vi "总磷总氮通讯.vi"() -> ()   [LabVIEW 2016, in "斯坦道总磷总氮.lvlib"]
uses:
  <vilib>/Plasmionique/MB Master/MB_Master_Serial/MB_Master_Serial.lvclass
  C:/Program Files (x86)/National Instruments/LabVIEW 2016/vi.lib/Plasmionique/MB Master/MB_Master/MB_Master.lvclass
  <vilib>/Plasmionique/MB Master/MB_Master_TCP/MB_Master_TCP.lvclass
  <vilib>/Utility/config.llb/Write Key (Boolean).vi
  <vilib>/Utility/config.llb/Write Key (String).vi
  <vilib>/Plasmionique/MB Master/MB_Master/MB_Master.lvclass
  <vilib>/Utility/config.llb/NI_LVConfig.lvlib
  <vilib>/Plasmionique/MB Master/MB Master.lvlib
  <vilib>/ptbypt/NI_PtbyPt.lvlib
panel:
  out "启用":bool=TRUE
  out "氨氮状态告警区":u16[](array[numeric])
  out "氨氮测量数据区":u16[](array[numeric])
  out "COD测量数据区":u16[](array[numeric])
  out "COD状态告警区":u16[](array[numeric])
  out "总氮测量数据区":u16[](array[numeric])
  out "总氮状态告警区":u16[](array[numeric])
  out "总磷状态告警区":u16[](array[numeric])
  out "总磷测量数据区":u16[](array[numeric])
  out "状态告警区":T1 {"告警代码" items=["无告警", "缺试剂告警", "缺水样告警", "缺蒸馏水告警", "缺标液告警", "仪表漏液告警", "标定异常告警", "超量程告警", "加热异常", "低试剂预警", "超上限告警", "超下限告警", "仪表内部其他异常", "滴定异常告警", "电极异常告警", "量程切换告警", "参数设置告警", "PH电极电位异常", "电导率电极异常", "浊度光度异常", "溶解氧电极异常", "溶解氧光强异常", "温度异常告警", "PH异常告警", "溶解氧异常告警", "电导率异常告警", "浊度异常告警", "叶绿素异常告警", "藻密度异常告警", "蓝绿藻异常告警", "ORP异常告警", "氨氮异常告警", "清洁刷异常告警", "SD卡异常告警", "蓝牙异常告警", "Wifi异常告警", "流程异常告警"]; "故障代码" items=["无故障", "电机故障", "温度故障", "通讯故障", "滴定故障"]}
  out "测量数据区":T2 {"单位" items=["ug/L", "mg/L", "ppm", "mg/m3", "cm", "ppb", "ug/m3", "%", "nmol/mol", "umol/mol", "MPN/L", "MPN/100ml", "ng/m3", "NTU", "无量纲", "ms/cm", "us/cm", "℃", "mV", "万个/L"]}
  out "status":bool
  out "关键参数区":T3
  in  "读关键参数区":bool
  in  "读状态告警区":bool
  in  "读测量数据区":bool
  in  "站号":u16(ring) items=["总磷"=1, "氨氮"=3]
  in  "停止":bool
  in  "启动":bool
  in  "控制命令":u16(ring) items=["启动测量"=1, "标样核查"=2, "零点核查"=3, "跨度核查"=4, "空白测试"=5, "平行样测试"=6, "加标回收"=7, "空白校准"=8, "标样校准"=9, "初始化（清洗）"=10, "停止测试"=11, "仪器重启"=12, "校时"=13, "模式设置"=14, "测量间隔设置"=15]
  in  "控制命令参数":u16[](array[numeric]) format="%04xH"
  in  "VISA Resource":refnum<visa-resource-name>
  in  "启用模块":bool
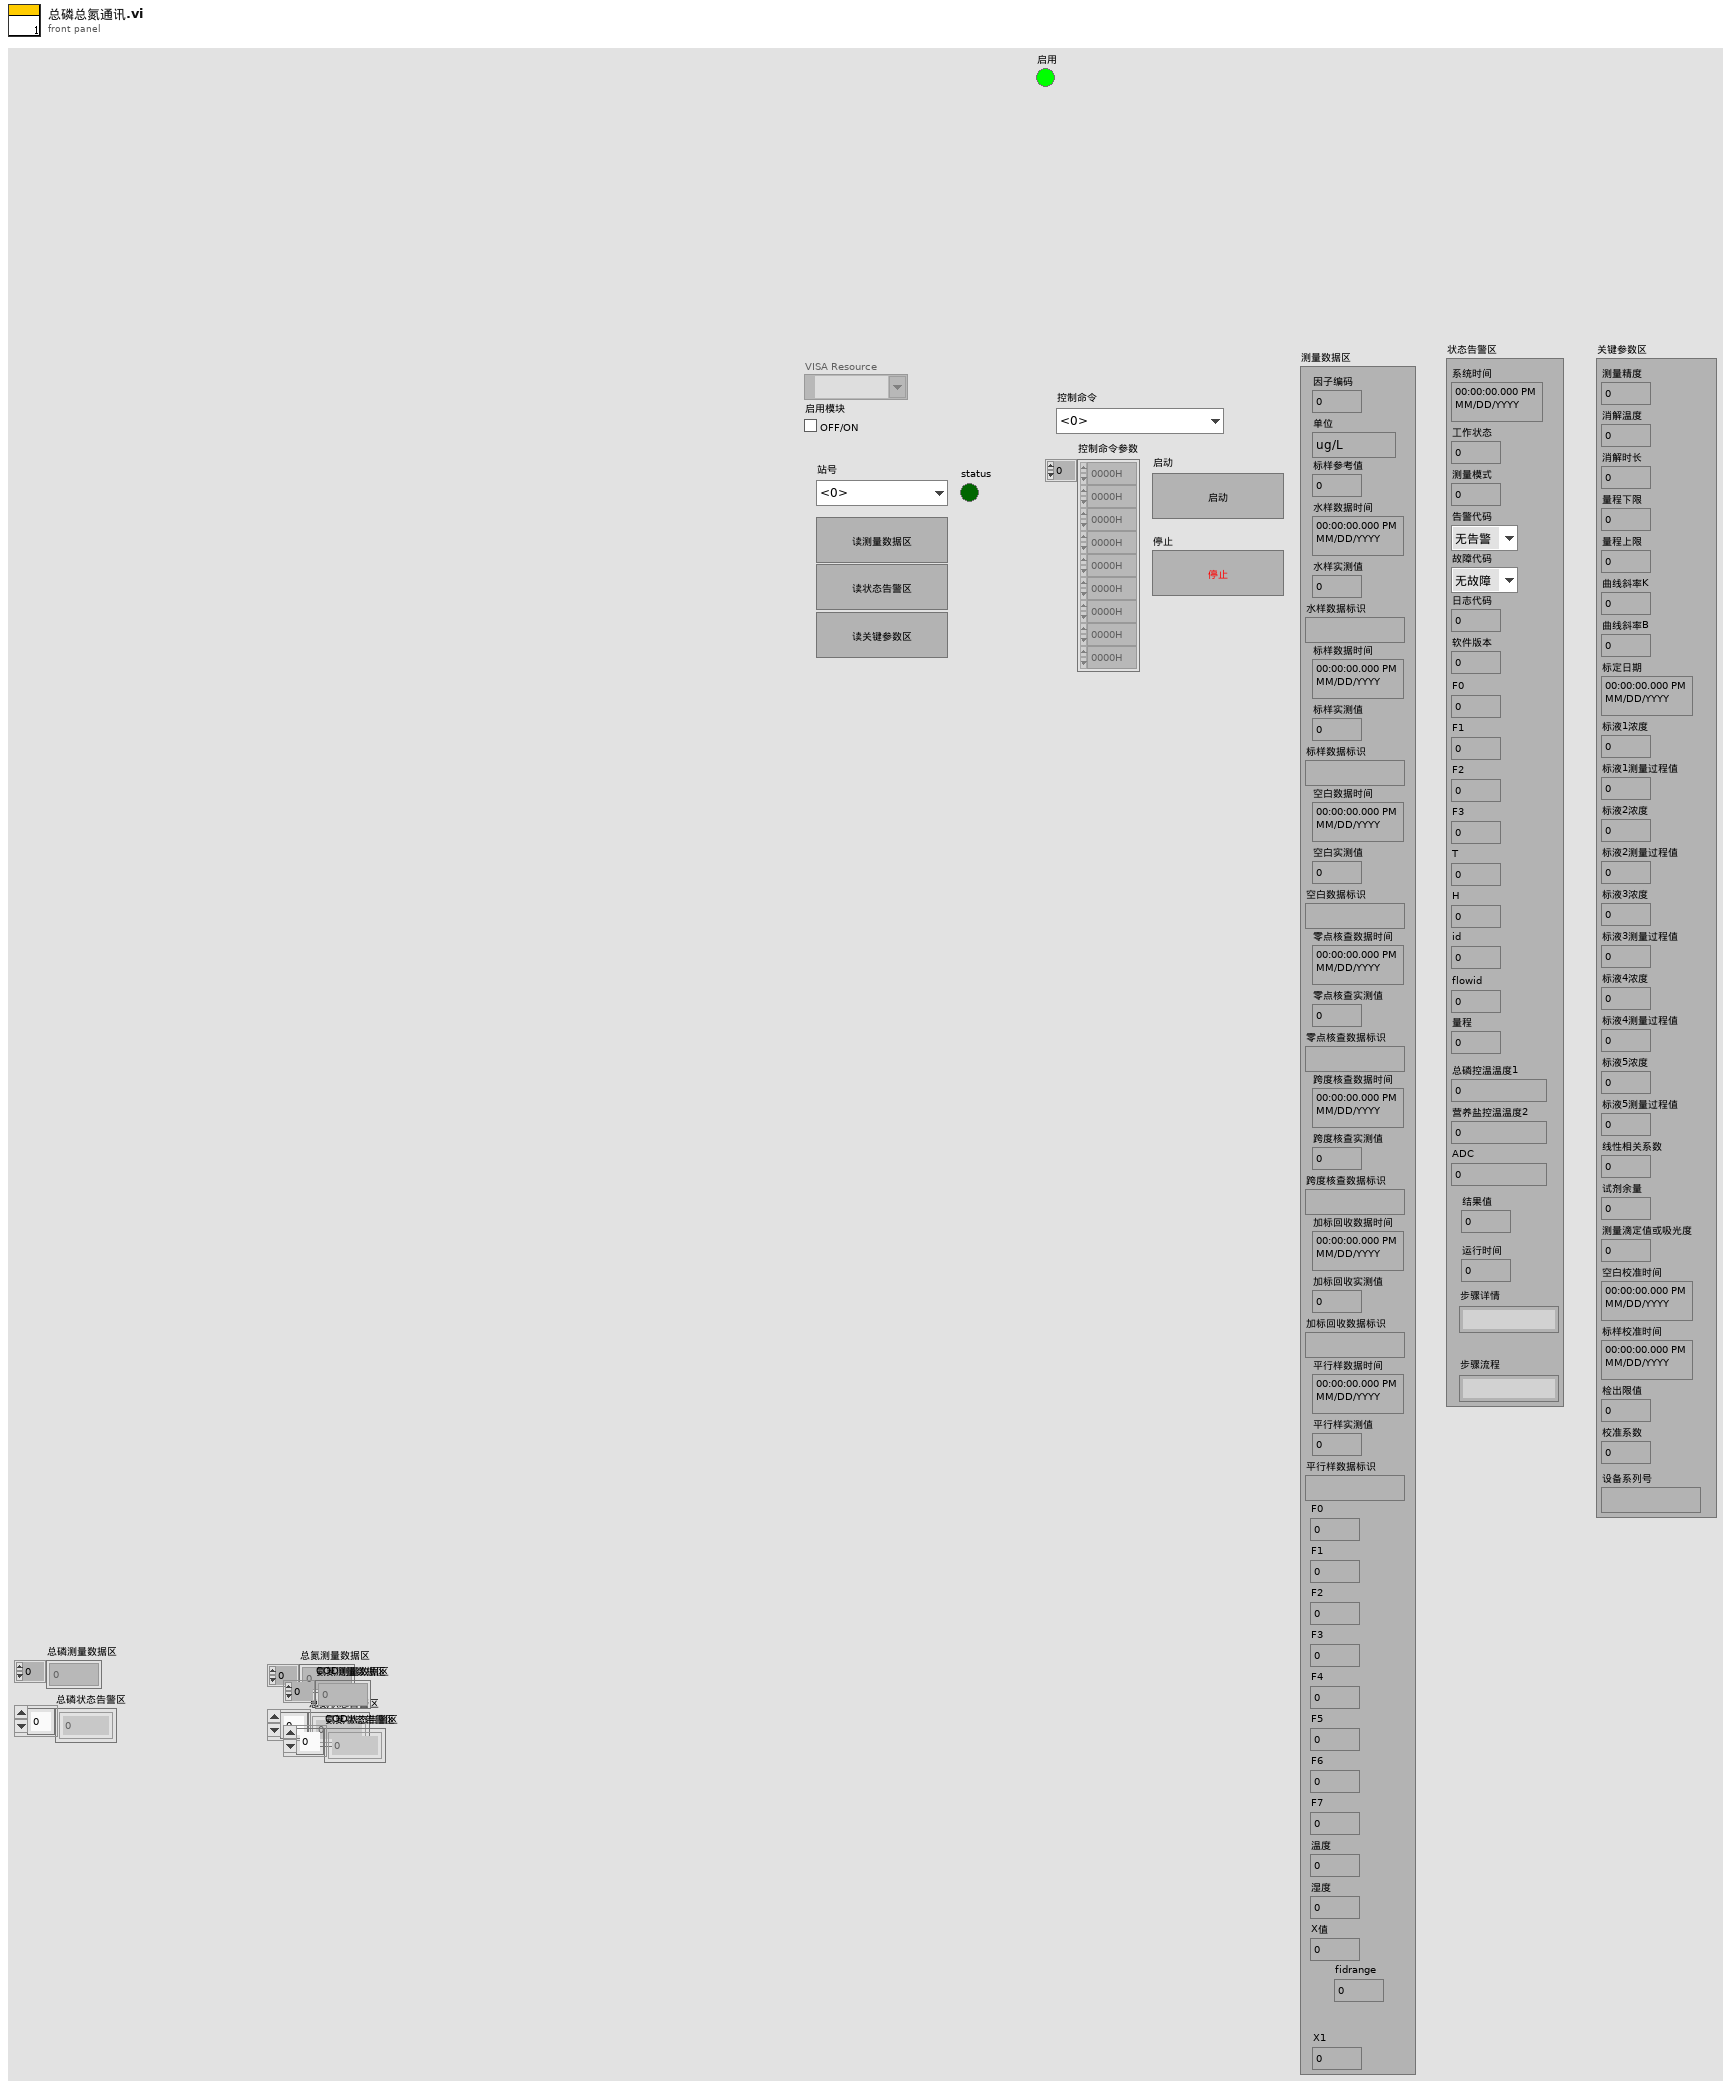
[diagram p1: front panel]
types:
  T1 = cluster{"系统时间":timestamp, "工作状态":u16, "测量模式":u16, "告警代码":u16, "故障代码":u16, "日志代码":u16, "软件版本":u16, "F0":sgl, "F1":sgl, "F2":sgl, "F3":sgl, "T":sgl, "H":sgl, "id":u16, "flowid":u16, "量程":u16, "总磷控温温度1":sgl, "营养盐控温温度2":sgl, "ADC":sgl, "结果值":sgl, "运行时间":u16, "步骤详情":string, "步骤流程":string}
  T2 = cluster{"因子编码":u32, "单位":u16, "标样参考值":sgl, "水样数据时间":timestamp, "水样实测值":sgl, "水样数据标识":string, "标样数据时间":timestamp, "标样实测值":sgl, "标样数据标识":string, "空白数据时间":timestamp, "空白实测值":sgl, "空白数据标识":string, "零点核查数据时间":timestamp, "零点核查实测值":sgl, "零点核查数据标识":string, "跨度核查数据时间":timestamp, "跨度核查实测值":sgl, "跨度核查数据标识":string, "加标回收数据时间":timestamp, "加标回收实测值":sgl, "加标回收数据标识":string, "平行样数据时间":timestamp, "平行样实测值":sgl, "平行样数据标识":string, "F0":sgl, "F1":sgl, "F2":sgl, "F3":sgl, "F4":sgl, "F5":sgl, "F6":sgl, "F7":sgl, "温度":sgl, "湿度":sgl, "X值":sgl, "fidrange":u16, "X1":sgl}
  T3 = cluster{"测量精度":u16, "消解温度":u16, "消解时长":u16, "量程下限":sgl, "量程上限":sgl, "曲线斜率K":sgl, "曲线斜率B":sgl, "标定日期":timestamp, "标液1浓度":sgl, "标液1测量过程值":sgl, "标液2浓度":sgl, "标液2测量过程值":sgl, "标液3浓度":sgl, "标液3测量过程值":sgl, "标液4浓度":sgl, "标液4测量过程值":sgl, "标液5浓度":sgl, "标液5测量过程值":sgl, "线性相关系数":sgl, "试剂余量":u32, "测量滴定值或吸光度":sgl, "空白校准时间":timestamp, "标样校准时间":timestamp, "检出限值":sgl, "校准系数":sgl, "设备系列号":string}
  T4 = cluster{"系统时间":timestamp, "工作状态":u16, "测量模式":enum16{"待机", "连续模式", "周期模式", "定点模式", "受控模式", "手动模式"}, "告警代码":u16, "故障代码":u16, "日志代码":u16, "软件版本":u16, "F0":sgl, "F1":sgl, "F2":sgl, "F3":sgl, "T":sgl, "H":sgl, "id":u16, "flowid":u16, "量程":u16, "总磷控温温度1":sgl, "营养盐控温温度2":sgl, "ADC":sgl}
  T5 = cluster{"因子编码":u32, "单位":u16, "标样参考值":sgl, "水样数据时间":timestamp, "水样实测值":sgl, "水样数据标识":string, "标样数据时间":timestamp, "标样实测值":sgl, "标样数据标识":string, "空白数据时间":timestamp, "空白实测值":sgl, "空白数据标识":string, "零点核查数据时间":timestamp, "零点核查实测值":sgl, "零点核查数据标识":string, "跨度核查数据时间":timestamp, "跨度核查实测值":sgl, "跨度核查数据标识":string, "加标回收数据时间":timestamp, "加标回收实测值":sgl, "加标回收数据标识":string, "平行样数据时间":timestamp, "平行样实测值":sgl, "平行样数据标识":string, "F0":sgl, "F1":sgl, "F2":sgl, "F3":sgl, "F4":sgl, "F5":sgl, "F6":sgl, "F7":sgl, "温度":sgl, "湿度":sgl, "X值":sgl, "fidrange":u16, "X1值":sgl}
  T6 = cluster{"测量精度":u16, "消解温度":u16, "消解时长":u16, "量程下限":sgl, "量程上限":sgl, "曲线斜率K":sgl, "曲线斜率B":sgl, "标定日期":timestamp, "标液1浓度":sgl, "标液1测量过程值":sgl, "标液2浓度":sgl, "标液2测量过程值":sgl, "标液3浓度":sgl, "标液3测量过程值":sgl, "标液4浓度":sgl, "标液4测量过程值":sgl, "标液5浓度":sgl, "标液5测量过程值":sgl, "线性相关系数":sgl, "试剂余量":u32, "测量滴定值或吸光度":sgl, "空白校准时间":timestamp, "标样校准时间":timestamp, "检出限值":sgl, "校准系数":sgl, "设备系列号":string}[]
  T7 = cluster{"系统时间":timestamp, "工作状态":u16, "测量模式":enum16{"待机", "连续模式", "周期模式", "定点模式", "受控模式", "手动模式"}, "告警代码":u16, "故障代码":u16, "日志代码":u16, "软件版本":u16, "F0":sgl, "F1":sgl, "F2":sgl, "F3":sgl, "T":sgl, "H":sgl, "id":u16, "flowid":u16, "量程":u16, "总磷控温温度1":sgl, "营养盐控温温度2":sgl, "ADC":sgl}[]
  T8 = cluster{"因子编码":u32, "单位":u16, "标样参考值":sgl, "水样数据时间":timestamp, "水样实测值":sgl, "水样数据标识":string, "标样数据时间":timestamp, "标样实测值":sgl, "标样数据标识":string, "空白数据时间":timestamp, "空白实测值":sgl, "空白数据标识":string, "零点核查数据时间":timestamp, "零点核查实测值":sgl, "零点核查数据标识":string, "跨度核查数据时间":timestamp, "跨度核查实测值":sgl, "跨度核查数据标识":string, "加标回收数据时间":timestamp, "加标回收实测值":sgl, "加标回收数据标识":string, "平行样数据时间":timestamp, "平行样实测值":sgl, "平行样数据标识":string, "F0":sgl, "F1":sgl, "F2":sgl, "F3":sgl, "F4":sgl, "F5":sgl, "F6":sgl, "F7":sgl, "温度":sgl, "湿度":sgl, "X值":sgl, "fidrange":u16, "X1值":sgl}[]
  T9 = enum16{"", "CODMn", "PH", "氨氮", "总氮", "总磷", "CODCr", "电导率", "水温", "溶解氧", "浊度", "叶绿素", "藻密度", "ORP"}
  T10 = typedef "CODCr交互.ctl" = cluster{"状态告警区":cluster{"系统时间":timestamp, "工作状态":u16, "测量模式":enum16{"待机", "连续模式", "周期模式", "定点模式", "受控模式", "手动模式"}, "告警代码":u16, "故障代码":u16, "日志代码":u16, "软件版本":u16, "F0":sgl, "F1":sgl, "F2":sgl, "F3":sgl, "T":sgl, "H":sgl, "id":u16, "flowid":u16, "量程":u16, "总磷控温温度1":sgl, "营养盐控温温度2":sgl, "ADC":sgl}, "平台试剂余量百分比":sgl, "关键参数":cluster{"测量量程":dbl, "测量精度":dbl, "测量间隔":dbl, "消解温度":dbl, "消解时长":dbl, "空白校准时间":timestamp, "曲线截距":dbl, "曲线斜率":dbl, "测量检出限":dbl, "测量信号值":dbl, "线性相关系数":dbl, "二次多项式系数":dbl, "标样校准时间":timestamp, "稀释倍数":dbl, "三项式系数":dbl, "空白标定系数":dbl, "量程系数":dbl, "F0/ORPA":dbl, "F1/ORPB":dbl, "F2/ORPK":dbl, "F3":dbl, "F4":dbl, "F5":dbl, "F6":dbl, "F7":dbl, "X0/滴定数":dbl, "量程":dbl}, "关键参数改变":bool, "校准信息":cluster{"低标液1浓度":dbl, "低标液1信号值":dbl, "低标液1启用":u16, "低标液2浓度":dbl, "低标液2信号值":dbl, "低标液2启用":u16, "低标液3浓度":dbl, "低标液3信号值":dbl, "低标液3启用":u16, "低标液4浓度":dbl, "低标液4信号值":dbl, "低标液4启用":u16, "低标液5浓度":dbl, "低标液5信号值":dbl, "低标液5启用":u16, "高标液1浓度":dbl, "高标液1信号值":dbl, "高标液1启用":u16, "高标液2浓度":dbl, "高标液2信号值":dbl, "高标液2启用":u16, "高标液3浓度":dbl, "高标液3信号值":dbl, "高标液3启用":u16, "高标液4浓度":dbl, "高标液4信号值":dbl, "高标液4启用":u16, "高标液5浓度":dbl, "高标液5信号值":dbl, "高标液5启用":u16, "低斜率":dbl, "低截距":dbl, "低二次多项式系数":dbl, "低线性相关系数":dbl, "高斜率":dbl, "高截距":dbl, "高二次多项式系数":dbl, "高线性相关系数":dbl}, "校准信息改变":bool, "固件版本号":string}
  T11 = typedef "氨氮交互.ctl" = cluster{"状态告警区":cluster{"系统时间":timestamp, "工作状态":u16, "测量模式":enum16{"待机", "连续模式", "周期模式", "定点模式", "受控模式", "手动模式"}, "告警代码":u16, "故障代码":u16, "日志代码":u16, "软件版本":u16, "F0":sgl, "F1":sgl, "F2":sgl, "F3":sgl, "T":sgl, "H":sgl, "id":u16, "flowid":u16, "量程":u16, "总磷控温温度1":sgl, "营养盐控温温度2":sgl, "ADC":sgl}, "平台试剂余量百分比":sgl, "关键参数":cluster{"测量量程":dbl, "测量精度":dbl, "测量间隔":dbl, "消解温度":dbl, "消解时长":dbl, "空白校准时间":timestamp, "曲线截距":dbl, "曲线斜率":dbl, "测量检出限":dbl, "测量信号值":dbl, "线性相关系数":dbl, "二次多项式系数":dbl, "标样校准时间":timestamp, "稀释倍数":dbl, "三项式系数":dbl, "空白标定系数":dbl, "量程系数":dbl, "F0/ORPA":dbl, "F1/ORPB":dbl, "F2/ORPK":dbl, "F3":dbl, "F4":dbl, "F5":dbl, "F6":dbl, "F7":dbl, "X0/滴定数":dbl, "量程":dbl}, "关键参数改变":bool, "校准信息":cluster{"低标液1浓度":dbl, "低标液1信号值":dbl, "低标液1启用":u16, "低标液2浓度":dbl, "低标液2信号值":dbl, "低标液2启用":u16, "低标液3浓度":dbl, "低标液3信号值":dbl, "低标液3启用":u16, "低标液4浓度":dbl, "低标液4信号值":dbl, "低标液4启用":u16, "低标液5浓度":dbl, "低标液5信号值":dbl, "低标液5启用":u16, "高标液1浓度":dbl, "高标液1信号值":dbl, "高标液1启用":u16, "高标液2浓度":dbl, "高标液2信号值":dbl, "高标液2启用":u16, "高标液3浓度":dbl, "高标液3信号值":dbl, "高标液3启用":u16, "高标液4浓度":dbl, "高标液4信号值":dbl, "高标液4启用":u16, "高标液5浓度":dbl, "高标液5信号值":dbl, "高标液5启用":u16, "低斜率":dbl, "低截距":dbl, "低二次多项式系数":dbl, "低线性相关系数":dbl, "高斜率":dbl, "高截距":dbl, "高二次多项式系数":dbl, "高线性相关系数":dbl}, "校准信息改变":bool, "固件版本号":string}
  T12 = typedef "总氮交互.ctl" = cluster{"状态告警区":cluster{"系统时间":timestamp, "工作状态":u16, "测量模式":enum16{"待机", "连续模式", "周期模式", "定点模式", "受控模式", "手动模式"}, "告警代码":u16, "故障代码":u16, "日志代码":u16, "软件版本":u16, "F0":sgl, "F1":sgl, "F2":sgl, "F3":sgl, "T":sgl, "H":sgl, "id":u16, "flowid":u16, "量程":u16, "总磷控温温度1":sgl, "营养盐控温温度2":sgl, "ADC":sgl}, "平台试剂余量百分比":sgl, "关键参数":cluster{"测量量程":dbl, "测量精度":dbl, "测量间隔":dbl, "消解温度":dbl, "消解时长":dbl, "空白校准时间":timestamp, "曲线截距":dbl, "曲线斜率":dbl, "测量检出限":dbl, "测量信号值":dbl, "线性相关系数":dbl, "二次多项式系数":dbl, "标样校准时间":timestamp, "稀释倍数":dbl, "三项式系数":dbl, "空白标定系数":dbl, "量程系数":dbl, "F0/ORPA":dbl, "F1/ORPB":dbl, "F2/ORPK":dbl, "F3":dbl, "F4":dbl, "F5":dbl, "F6":dbl, "F7":dbl, "X0/滴定数":dbl, "量程":dbl}, "关键参数改变":bool, "校准信息":cluster{"低标液1浓度":dbl, "低标液1信号值":dbl, "低标液1启用":u16, "低标液2浓度":dbl, "低标液2信号值":dbl, "低标液2启用":u16, "低标液3浓度":dbl, "低标液3信号值":dbl, "低标液3启用":u16, "低标液4浓度":dbl, "低标液4信号值":dbl, "低标液4启用":u16, "低标液5浓度":dbl, "低标液5信号值":dbl, "低标液5启用":u16, "高标液1浓度":dbl, "高标液1信号值":dbl, "高标液1启用":u16, "高标液2浓度":dbl, "高标液2信号值":dbl, "高标液2启用":u16, "高标液3浓度":dbl, "高标液3信号值":dbl, "高标液3启用":u16, "高标液4浓度":dbl, "高标液4信号值":dbl, "高标液4启用":u16, "高标液5浓度":dbl, "高标液5信号值":dbl, "高标液5启用":u16, "低斜率":dbl, "低截距":dbl, "低二次多项式系数":dbl, "低线性相关系数":dbl, "高斜率":dbl, "高截距":dbl, "高二次多项式系数":dbl, "高线性相关系数":dbl}, "校准信息改变":bool, "固件版本号":string}
  T13 = typedef "总磷交互.ctl" = cluster{"状态告警区":cluster{"系统时间":timestamp, "工作状态":u16, "测量模式":enum16{"待机", "连续模式", "周期模式", "定点模式", "受控模式", "手动模式"}, "告警代码":u16, "故障代码":u16, "日志代码":u16, "软件版本":u16, "F0":sgl, "F1":sgl, "F2":sgl, "F3":sgl, "T":sgl, "H":sgl, "id":u16, "flowid":u16, "量程":u16, "总磷控温温度1":sgl, "营养盐控温温度2":sgl, "ADC":sgl}, "平台试剂余量百分比":sgl, "关键参数":cluster{"测量量程":dbl, "测量精度":dbl, "测量间隔":dbl, "消解温度":dbl, "消解时长":dbl, "空白校准时间":timestamp, "曲线截距":dbl, "曲线斜率":dbl, "测量检出限":dbl, "测量信号值":dbl, "线性相关系数":dbl, "二次多项式系数":dbl, "标样校准时间":timestamp, "稀释倍数":dbl, "三项式系数":dbl, "空白标定系数":dbl, "量程系数":dbl, "F0/ORPA":dbl, "F1/ORPB":dbl, "F2/ORPK":dbl, "F3":dbl, "F4":dbl, "F5":dbl, "F6":dbl, "F7":dbl, "X0/滴定数":dbl, "量程":dbl}, "关键参数改变":bool, "校准信息":cluster{"低标液1浓度":dbl, "低标液1信号值":dbl, "低标液1启用":u16, "低标液2浓度":dbl, "低标液2信号值":dbl, "低标液2启用":u16, "低标液3浓度":dbl, "低标液3信号值":dbl, "低标液3启用":u16, "低标液4浓度":dbl, "低标液4信号值":dbl, "低标液4启用":u16, "低标液5浓度":dbl, "低标液5信号值":dbl, "低标液5启用":u16, "高标液1浓度":dbl, "高标液1信号值":dbl, "高标液1启用":u16, "高标液2浓度":dbl, "高标液2信号值":dbl, "高标液2启用":u16, "高标液3浓度":dbl, "高标液3信号值":dbl, "高标液3启用":u16, "高标液4浓度":dbl, "高标液4信号值":dbl, "高标液4启用":u16, "高标液5浓度":dbl, "高标液5信号值":dbl, "高标液5启用":u16, "低斜率":dbl, "低截距":dbl, "低二次多项式系数":dbl, "低线性相关系数":dbl, "高斜率":dbl, "高截距":dbl, "高二次多项式系数":dbl, "高线性相关系数":dbl}, "校准信息改变":bool, "固件版本号":string}
  T14 = typedef "操作日志字段定义.ctl" = cluster{"时间":timestamp, "参数":string, "日志信息":string, "流程参数":string}
  T15 = typedef "NI_LVConfig.lvlib/Config Data RefNum.ctl" = refnum<k1>
  T16 = enum8{"Enabled", "Disabled", "Disabled and Grayed Out"}
  T17 = cluster{"baud rate (bps)":u32, "stop bits":u16, "parity":u16, "flow control":u16, "timeout":u32, "retries":i32}
  T18 = typedef "工况数据.ctl" = cluster{"time":string, "data":cluster{"ups":cluster{"ups":cluster{"input_voltage":ext, "input_frequency":ext, "output_voltage":ext, "output_current":ext, "output_frequency":ext, "output_active_power":ext, "output_apparent_power":ext, "load_rate":ext, "cabinet_temperature":ext, "battery_voltage":ext, "remaining_battery_capacity":ext, "power_on_status":string, "power_supply_mode":string, "fault":bool, "battery_low_voltage":bool, "mains_supply_abnormality":bool}, "启用":bool}, "air_conditioner":cluster{"air_conditioner":cluster{"cabinet_temperature":ext, "air_supply_temperature":ext, "voltage":ext, "current":ext, "compressor_status":string, "Internal_fan_status":string, "external_fan_status":string, "heating_state":string, "refrigeration_state":bool, "high_temperature_alarm":bool, "low_temperature_alarm":bool, "heater_fault":bool, "temperature_sensor_fault":bool, "high_voltage_alarm":bool, "low_voltage_alarm":bool, "refrigeration_start_point":ext, "refrigeration_sensitive_point":ext, "heating_start_point":ext, "heating_sensitive_point":ext, "high_temperature_alarm_point":ext, "low_temperature_alarm_point":ext}, "启用":bool}, "smoke_sensor":cluster{"smoke_sensor":cluster{"trigger_alarm":bool}, "启用":bool}, "water_immersion_sensor":cluster{"water_immersion_sensor":cluster{"trigger_alarm":bool}, "启用":bool}, "temperature_and_humidity_sensor":cluster{"temperature_and_humidity_sensor":cluster{"current_temperature":ext, "current_humidity":ext, "room_temperature_alarm":bool, "humidity_alarm":bool}, "启用":bool}, "gps":cluster{"gps":cluster{"current_longitude":ext, "current_latitude":ext, "launch_longitude":ext, "launch_latitude":ext, "shift_alarm":bool}, "启用":bool}, "solar_controller":cluster{"solar_controller":cluster{"array_voltage":ext, "array_current":ext, "generating_power":ext, "battery_voltage":dbl, "battery_current":ext, "ceiling_voltage":ext, "minimum_voltage":ext, "battery_temperature":ext, "remaining_battery_capacity":ext, "load_voltage":ext, "load_current":ext, "load_power":ext, "equipment_temperature":ext, "accumulated_electricity_consumption_of_the_day":ext, "accumulated_electricity_consumption_of_the_current_month":ext, "accumulated_electricity_consumption_in_the_current_year":ext, "total_accumulated_power_consumption":ext, "accumulated_charging_capacity_of_the_day":ext, "accumulated_charging_amount_of_the_current_month":ext, "accumulated_charging_capacity_of_the_current_year":ext, "total_cumulative_charge":ext}, "启用":bool}, "solar_controller_2":cluster{"solar_controller_2":cluster{"array_voltage":ext, "array_current":ext, "generating_power":ext, "battery_voltage":dbl, "battery_current":ext, "ceiling_voltage":ext, "minimum_voltage":ext, "battery_temperature":ext, "remaining_battery_capacity":ext, "load_voltage":ext, "load_current":ext, "load_power":ext, "equipment_temperature":ext, "accumulated_electricity_consumption_of_the_day":ext, "accumulated_electricity_consumption_of_the_current_month":ext, "accumulated_electricity_consumption_in_the_current_year":ext, "total_accumulated_power_consumption":ext, "accumulated_charging_capacity_of_the_day":ext, "accumulated_charging_amount_of_the_current_month":ext, "accumulated_charging_capacity_of_the_current_year":ext, "total_cumulative_charge":ext}, "启用":bool}, "NH3":cluster{"NH3":cluster{"F0":ext, "F1":ext, "syringe_temperature":ext, "alarm_step":dbl, "X0":ext}, "启用":bool}, "TP":cluster{"TP":cluster{"F0":ext, "F1":ext, "F2":ext, "F3":ext, "digestion_temperature":ext, "constant_temperature":ext, "syringe_temperature":ext, "alarm_step":dbl, "X0":ext}, "启用":bool}, "TN":cluster{"TN":cluster{"F0":ext, "F1":ext, "F2":ext, "F3":ext, "F4":ext, "F5":ext, "F6":ext, "F7":ext, "digestion_temperature":ext, "constant_temperature":ext, "syringe_temperature":ext, "alarm_step":dbl, "X0":ext}, "启用":bool}, "CODMn":cluster{"CODMn":cluster{"temperature_curve":ext[], "titration_curve":ext[], "F0":ext, "F1":ext, "F2":ext, "F3":ext, "F4":ext, "F5":ext, "A":ext, "B":ext, "K":ext}, "启用":bool}, "CODCr":cluster{"CODCr":cluster{"temperature_curve":ext[], "F0":ext, "F1":ext, "reagent_sensor":ext}, "启用":bool}}}
  T19 = cluster{"系统时间":timestamp, "工作状态":u16, "测量模式":enum16{"待机", "连续模式", "周期模式", "定点模式", "受控模式", "手动模式"}, "告警代码":u16, "故障代码":u16, "日志代码":u16, "软件版本":u16, "F0":sgl, "F1":sgl, "F2":sgl, "F3":sgl, "T":sgl, "H":sgl, "id":u16, "flowid":u16, "量程":u16, "总磷控温温度1":sgl, "营养盐控温温度2":sgl, "ADC":sgl, "结果值":sgl, "运行时间":u16, "步骤详情":string, "步骤流程":string}
  T20 = typedef "斯坦道总磷总氮.lvlib/关键参数.ctl" = cluster{"测量量程":sgl, "测量检出限":sgl, "测量精度":sgl, "测量间隔":sgl, "消解温度":sgl, "消解时长":sgl, "三项式系数":sgl, "二次多项式系数":sgl, "曲线斜率":sgl, "曲线截距":sgl, "线性相关系数":sgl, "空白校准时间":timestamp, "标样校准时间":timestamp, "测量信号值":sgl, "稀释倍数":sgl, "空白标定系数":sgl, "量程系数":sgl}
  T21 = cluster{"测量量程":dbl, "测量精度":dbl, "测量间隔":dbl, "消解温度":dbl, "消解时长":dbl, "空白校准时间":timestamp, "曲线截距":dbl, "曲线斜率":dbl, "测量检出限":dbl, "测量信号值":dbl, "线性相关系数":dbl, "二次多项式系数":dbl, "标样校准时间":timestamp, "稀释倍数":dbl, "三项式系数":dbl, "空白标定系数":dbl, "量程系数":dbl, "F0/ORPA":dbl, "F1/ORPB":dbl, "F2/ORPK":dbl, "F3":dbl, "F4":dbl, "F5":dbl, "F6":dbl, "F7":dbl, "X0/滴定数":dbl, "量程":dbl}
  T22 = cluster{"低标液1浓度":dbl, "低标液1信号值":dbl, "低标液1启用":u16, "低标液2浓度":dbl, "低标液2信号值":dbl, "低标液2启用":u16, "低标液3浓度":dbl, "低标液3信号值":dbl, "低标液3启用":u16, "低标液4浓度":dbl, "低标液4信号值":dbl, "低标液4启用":u16, "低标液5浓度":dbl, "低标液5信号值":dbl, "低标液5启用":u16, "高标液1浓度":dbl, "高标液1信号值":dbl, "高标液1启用":u16, "高标液2浓度":dbl, "高标液2信号值":dbl, "高标液2启用":u16, "高标液3浓度":dbl, "高标液3信号值":dbl, "高标液3启用":u16, "高标液4浓度":dbl, "高标液4信号值":dbl, "高标液4启用":u16, "高标液5浓度":dbl, "高标液5信号值":dbl, "高标液5启用":u16, "低斜率":dbl, "低截距":dbl, "低二次多项式系数":dbl, "低线性相关系数":dbl, "高斜率":dbl, "高截距":dbl, "高二次多项式系数":dbl, "高线性相关系数":dbl}
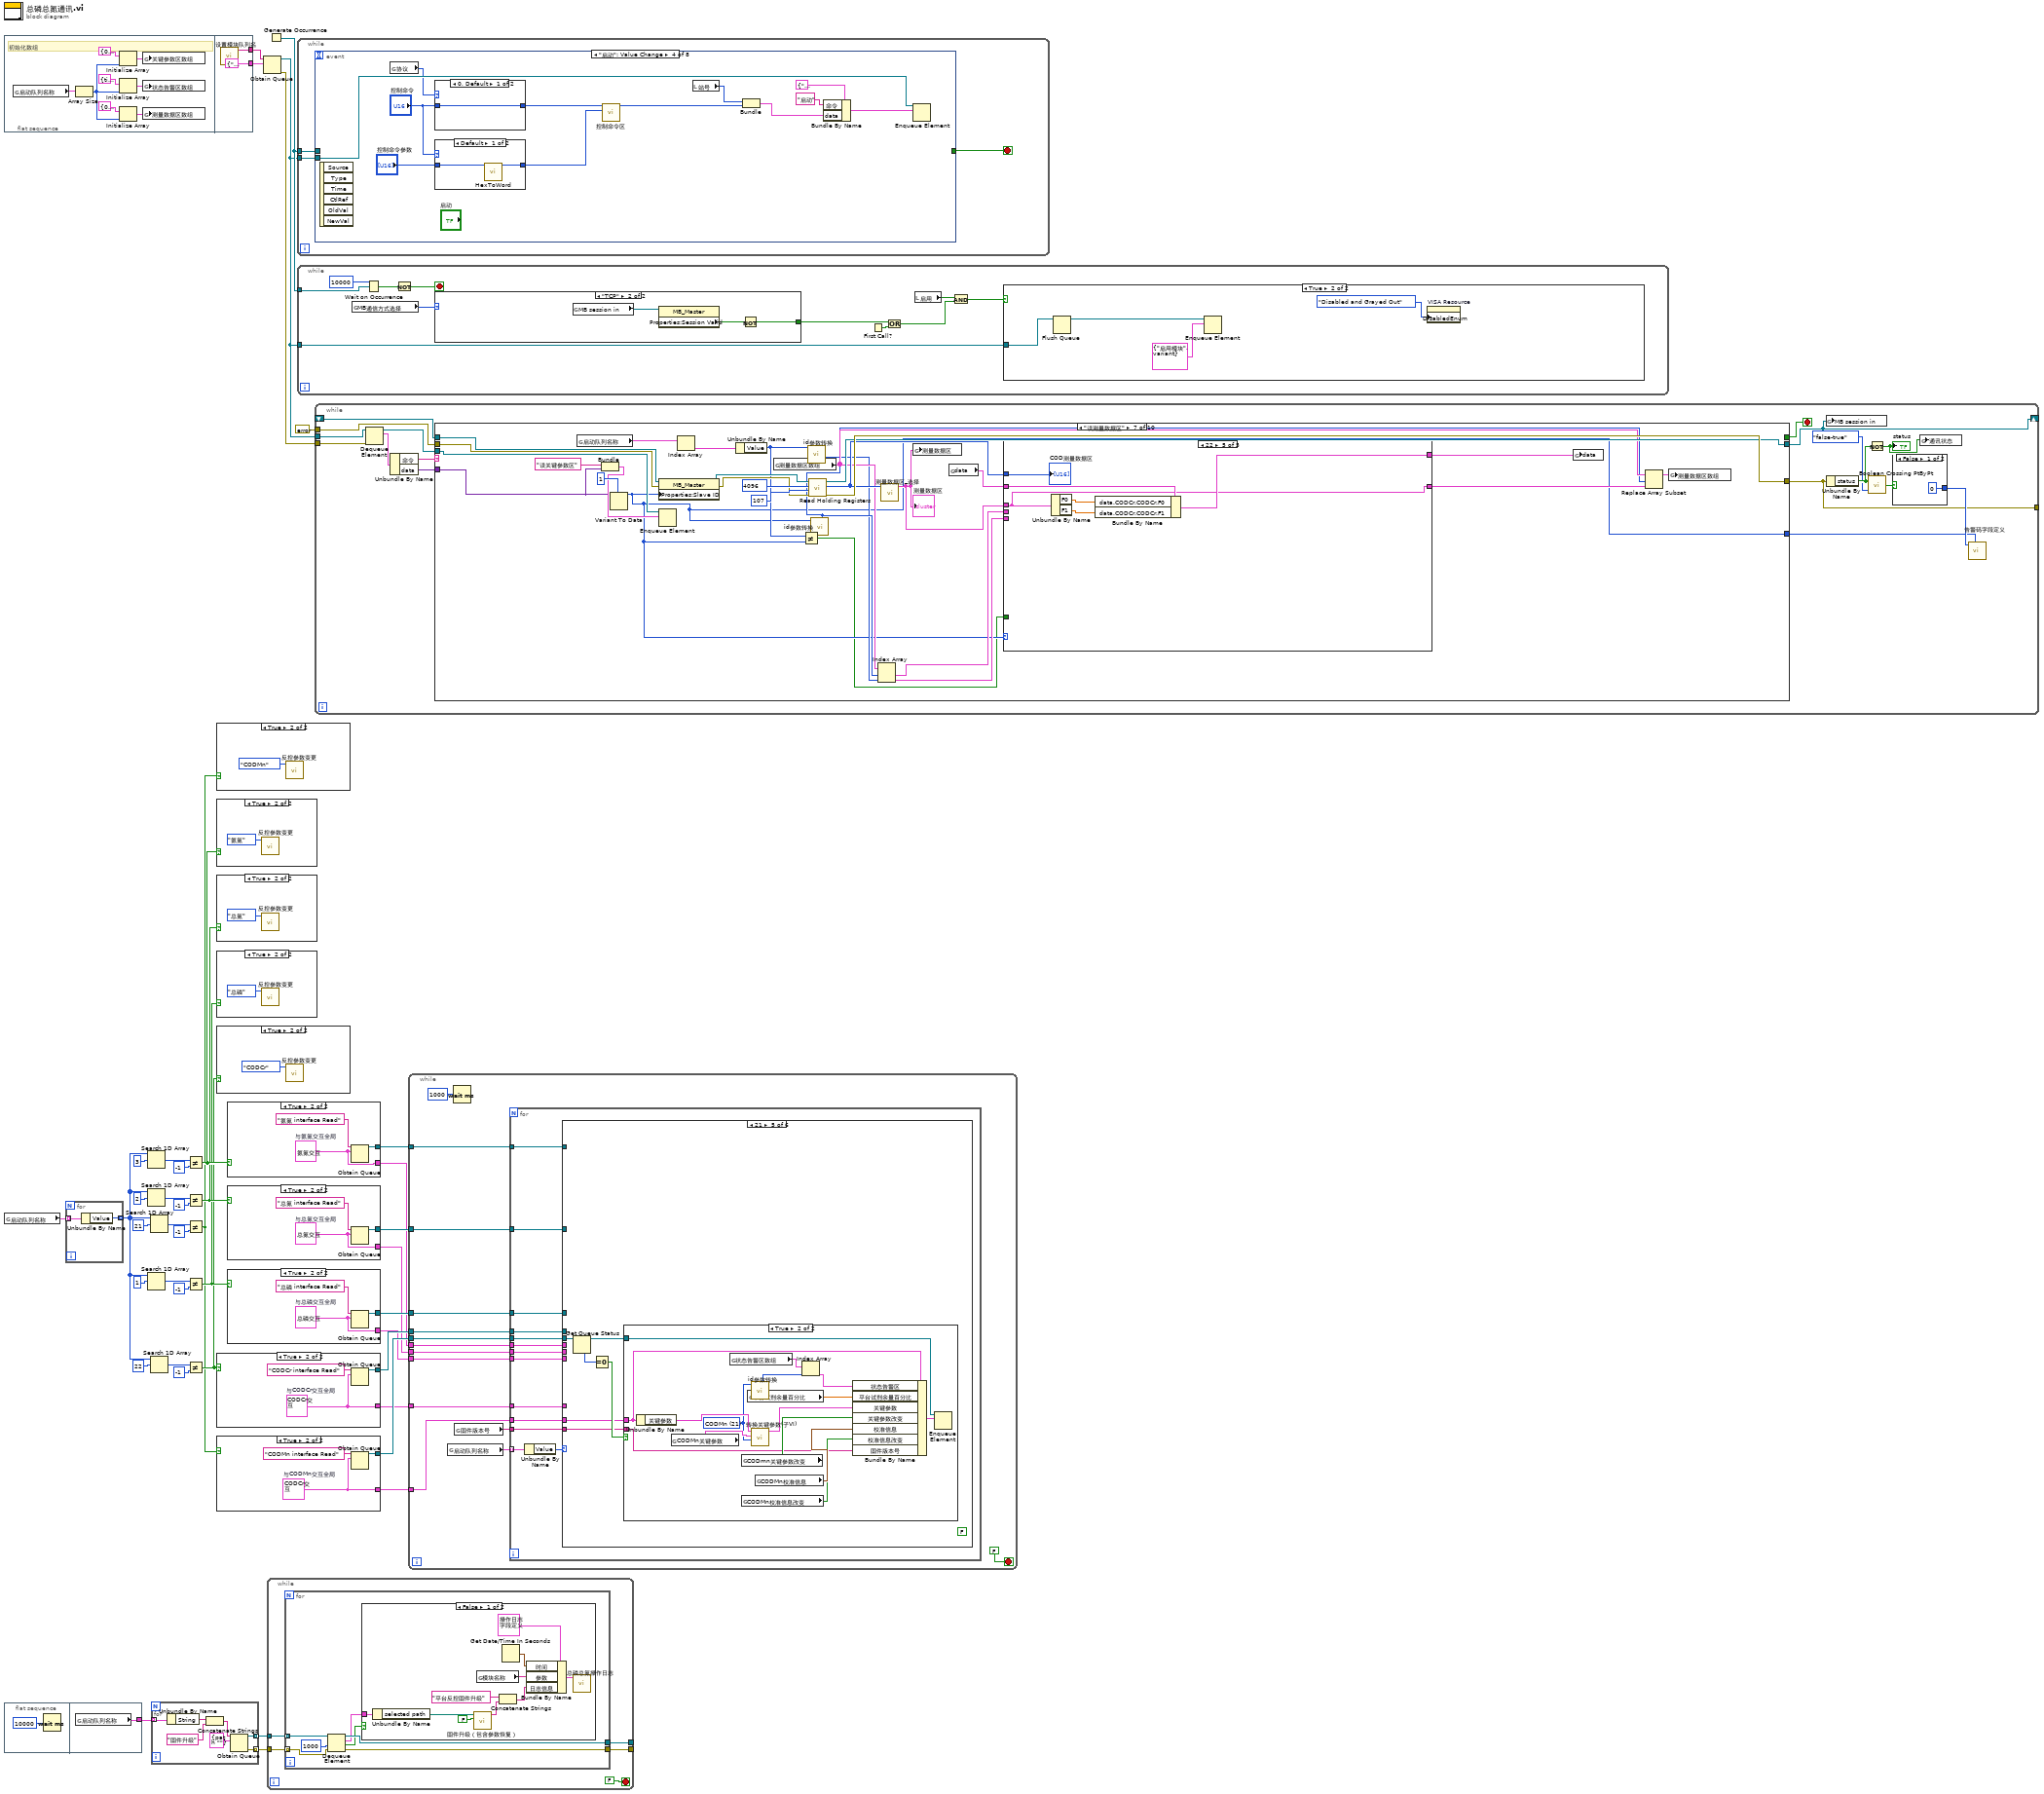
[diagram p0: block diagram]
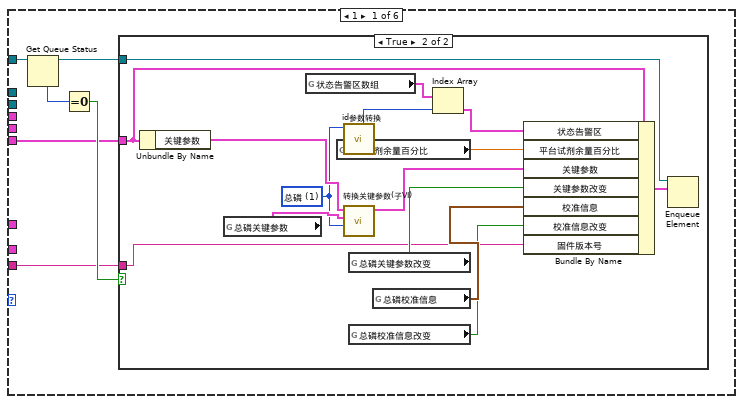
[diagram p13: hidden frame]
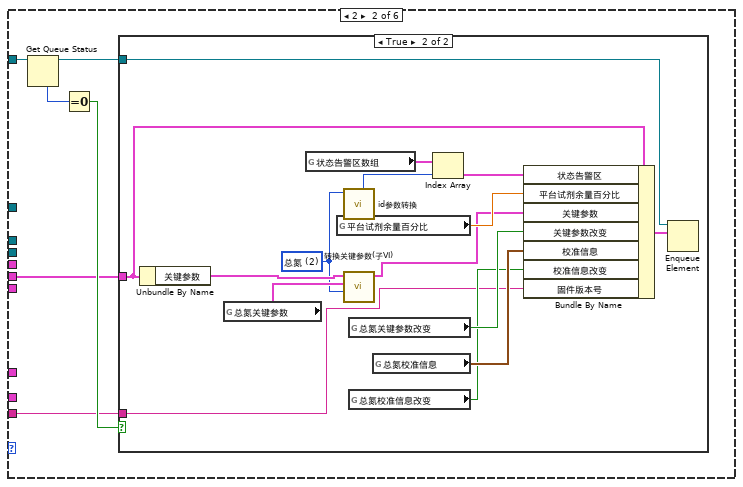
[diagram p15: hidden frame]
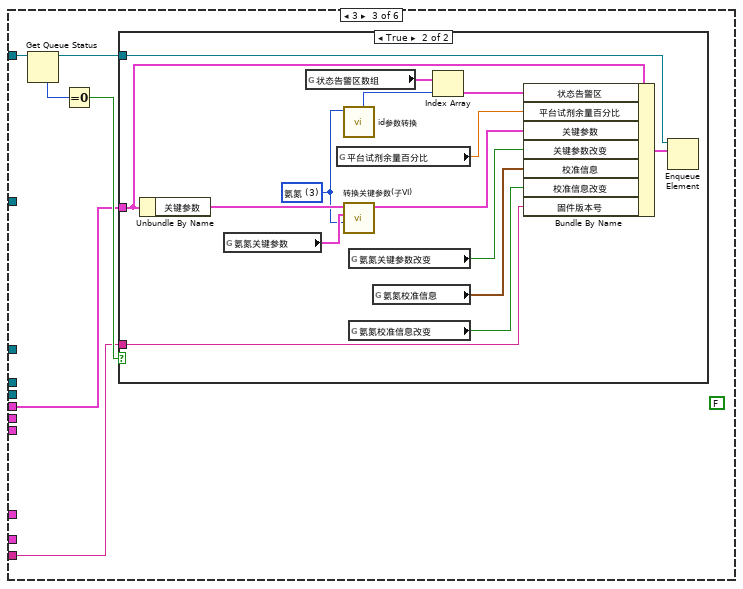
[diagram p17: hidden frame]
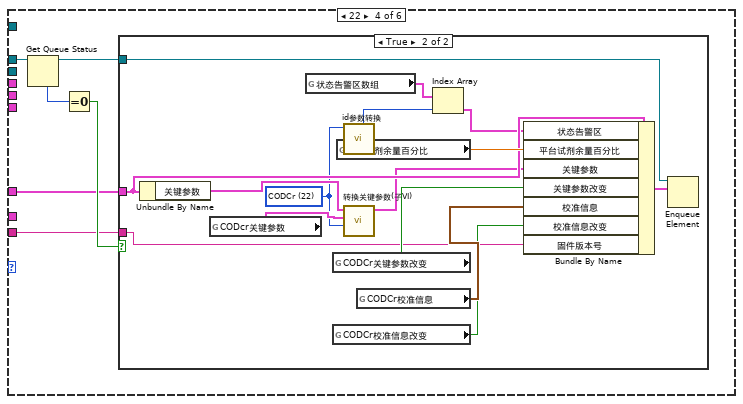
[diagram p19: hidden frame]
diagram:
  n1 = flat-sequence {
    tunnel: [cluster{"命令":string, "data":variant} {"命令"="", "data"=variant}] -> w41
    tunnel: [w50] -> w36
    frame #0 {
      # "初始化数组"
      n2 = global read "model config var.vi" "启动队列名称"() -> (w43:cluster{"String":string, "Value":u16}[])
      n3 = Array Size(array=w43) -> (size(s)=w42:i32)
      n4 = Initialize Array(T3 {"测量精度"=0, "消解温度"=0, "消解时长"=0, "量程下限"=0.0, "量程上限"=0.0, "曲线斜率K"=0.0, "曲线斜率B"=0.0, "标定日期"=timestamp(0 s since 1904-01-01), "标液1浓度"=0.0, "标液1测量过程值"=0.0, "标液2浓度"=0.0, "标液2测量过程值"=0.0, "标液3浓度"=0.0, "标液3测量过程值"=0.0, "标液4浓度"=0.0, "标液4测量过程值"=0.0, "标液5浓度"=0.0, "标液5测量过程值"=0.0, "线性相关系数"=0.0, "试剂余量"=0, "测量滴定值或吸光度"=0.0, "空白校准时间"=timestamp(0 s since 1904-01-01), "标样校准时间"=timestamp(0 s since 1904-01-01), "检出限值"=0.0, "校准系数"=0.0, "设备系列号"=""} ("关键参数区"), w42) -> (w47:T6)
      n5 = Initialize Array(T4 {"系统时间"=timestamp(0 s since 1904-01-01), "工作状态"=0, "测量模式"=enum."待机", "告警代码"=0, "故障代码"=0, "日志代码"=0, "软件版本"=0, "F0"=0.0, "F1"=0.0, "F2"=0.0, "F3"=0.0, "T"=0.0, "H"=0.0, "id"=0, "flowid"=0, "量程"=0, "总磷控温温度1"=0.0, "营养盐控温温度2"=0.0, "ADC"=0.0} ("状态告警区"), w42) -> (w46:T7)
      n6 = Initialize Array(T5 {"因子编码"=0, "单位"=0, "标样参考值"=0.0, "水样数据时间"=timestamp(0 s since 1904-01-01), "水样实测值"=0.0, "水样数据标识"="", "标样数据时间"=timestamp(0 s since 1904-01-01), "标样实测值"=0.0, "标样数据标识"="", "空白数据时间"=timestamp(0 s since 1904-01-01), "空白实测值"=0.0, "空白数据标识"="", "零点核查数据时间"=timestamp(0 s since 1904-01-01), "零点核查实测值"=0.0, "零点核查数据标识"="", "跨度核查数据时间"=timestamp(0 s since 1904-01-01), "跨度核查实测值"=0.0, "跨度核查数据标识"="", "加标回收数据时间"=timestamp(0 s since 1904-01-01), "加标回收实测值"=0.0, "加标回收数据标识"="", "平行样数据时间"=timestamp(0 s since 1904-01-01), "平行样实测值"=0.0, "平行样数据标识"="", "F0"=0.0, "F1"=0.0, "F2"=0.0, "F3"=0.0, "F4"=0.0, "F5"=0.0, "F6"=0.0, "F7"=0.0, "温度"=0.0, "湿度"=0.0, "X值"=0.0, "fidrange"=0, "X1值"=0.0} ("测量数据区"), w42) -> (w49:T8)
      n7 = global write "VAR总磷总氮全局变量.vi" "关键参数区数组"(w47) -> ()
      n8 = global write "VAR总磷总氮全局变量.vi" "状态告警区数组"(w46) -> ()
      n9 = global write "VAR总磷总氮全局变量.vi" "测量数据区数组"(w49) -> ()
    }
    frame #1 {
      n10 = call "设置模块队列名.vi"() -> ("Msg"=w50:string)  [unwired: 5 in]
    }
  }
  n11 = global read "model config var.vi" "启动队列名称"() -> (w25:cluster{"String":string, "Value":u16}[])
  n12 = flat-sequence {
    tunnel: [w53] -> w8
    frame #0 {
      n13 = Wait (ms)(milliseconds to wait=u32 10000 ("等待时间（毫秒）")) -> ()  [unwired: 1 out]
    }
    frame #1 {
      n14 = global read "model config var.vi" "启动队列名称"() -> (w53:cluster{"String":string, "Value":u16}[])
    }
  }
  n15 = for {
    tunnel: w25 -> [w55] mode=indexing
    tunnel: [w54] -> w9 mode=indexing
    n16 = Unbundle By Name(w55) -> ("Value"=w54:u16)
  }
  n17 = Search 1D Array(1D array=w9, element=u16 3 ("元素")) -> (index of element=w11:i32)  [unwired: 1 in]
  n18 = Search 1D Array(1D array=w9, element=u16 2 ("元素")) -> (index of element=w14:i32)  [unwired: 1 in]
  n19 = Search 1D Array(1D array=w9, element=u16 1 ("元素")) -> (index of element=w17:i32)  [unwired: 1 in]
  n20 = Search 1D Array(1D array=w9, element=u16 21 ("元素")) -> (index of element=w23:i32)  [unwired: 1 in]
  n21 = Search 1D Array(1D array=w9, element=u16 22 ("元素")) -> (index of element=w20:i32)  [unwired: 1 in]
  n22 = for {
    tunnel: w8 -> [w62] mode=indexing
    tunnel: [w57] -> w7 mode=indexing
    tunnel: [w56] -> w6 mode=indexing
    n23 = Unbundle By Name(w62) -> ("String"=w58:string)
    n24 = Concatenate Strings(w58, "固件升级" ("字符串")) -> (w60:string)
    n25 = Obtain Queue(name (unnamed)=w60, element data type=cluster{"selected path":path} {"selected path"=path ""}) -> (queue out=w57:refnum<queue>, error out=w56:errorcluster)  [unwired: 3 in, 1 out]
  }
  n26 = Not Equal?(x=w11, y=-1) -> (x != y?=w5:bool)
  n27 = Not Equal?(x=w14, y=-1) -> (x != y?=w4:bool)
  n28 = Not Equal?(x=w23, y=-1) -> (x != y?=w1:bool)
  n29 = Not Equal?(x=w17, y=-1) -> (x != y?=w3:bool)
  n30 = Not Equal?(x=w20, y=-1) -> (x != y?=w2:bool)
  n31 = case shown="True" w1 {
    frame False {
    }
    frame True {
      n32 = call "反控参数变更.vi"("设置参数"=T9."CODMn") -> ()  [unwired: 11 in]
    }
  }
  n33 = case shown="True" w5 {
    frame False {
    }
    frame True {
      n34 = call "反控参数变更.vi"("设置参数"=T9."氨氮") -> ()  [unwired: 11 in]
    }
  }
  n35 = case shown="True" w4 {
    frame False {
    }
    frame True {
      n36 = call "反控参数变更.vi"("设置参数"=T9."总氮") -> ()  [unwired: 11 in]
    }
  }
  n37 = case shown="True" w3 {
    frame False {
    }
    frame True {
      n38 = call "反控参数变更.vi"("设置参数"=T9."总磷") -> ()  [unwired: 11 in]
    }
  }
  n39 = case shown="True" w2 {
    frame False {
    }
    frame True {
      n40 = call "反控参数变更.vi"("设置参数"=T9."CODCr") -> ()  [unwired: 11 in]
    }
  }
  n41 = case shown="True" w2 {
    tunnel: [_ w69] -> w33
    tunnel: [_ w68] -> w32
    frame False {
    }
    frame True {
      w68 = T10 {"状态告警区"={"系统时间"=timestamp(0 s since 1904-01-01), "工作状态"=0, "测量模式"=enum."待机", "告警代码"=0, "故障代码"=0, "日志代码"=0, "软件版本"=0, "F0"=0.0, "F1"=0.0, "F2"=0.0, "F3"=0.0, "T"=0.0, "H"=0.0, "id"=0, "flowid"=0, "量程"=0, "总磷控温温度1"=0.0, "营养盐控温温度2"=0.0, "ADC"=0.0}, "平台试剂余量百分比"=0.0, "关键参数"={"测量量程"=0.0, "测量精度"=0.0, "测量间隔"=0.0, "消解温度"=0.0, "消解时长"=0.0, "空白校准时间"=timestamp(0 s since 1904-01-01), "曲线截距"=0.0, "曲线斜率"=0.0, "测量检出限"=0.0, "测量信号值"=0.0, "线性相关系数"=0.0, "二次多项式系数"=0.0, "标样校准时间"=timestamp(0 s since 1904-01-01), "稀释倍数"=0.0, "三项式系数"=0.0, "空白标定系数"=0.0, "量程系数"=0.0, "F0/ORPA"=0.0, "F1/ORPB"=0.0, "F2/ORPK"=0.0, "F3"=0.0, "F4"=0.0, "F5"=0.0, "F6"=0.0, "F7"=0.0, "X0/滴定数"=0.0, "量程"=0.0}, "关键参数改变"=FALSE, "校准信息"={"低标液1浓度"=0.0, "低标液1信号值"=0.0, "低标液1启用"=0, "低标液2浓度"=0.0, "低标液2信号值"=0.0, "低标液2启用"=0, "低标液3浓度"=0.0, "低标液3信号值"=0.0, "低标液3启用"=0, "低标液4浓度"=0.0, "低标液4信号值"=0.0, "低标液4启用"=0, "低标液5浓度"=0.0, "低标液5信号值"=0.0, "低标液5启用"=0, "高标液1浓度"=0.0, "高标液1信号值"=0.0, "高标液1启用"=0, "高标液2浓度"=0.0, "高标液2信号值"=0.0, "高标液2启用"=0, "高标液3浓度"=0.0, "高标液3信号值"=0.0, "高标液3启用"=0, "高标液4浓度"=0.0, "高标液4信号值"=0.0, "高标液4启用"=0, "高标液5浓度"=0.0, "高标液5信号值"=0.0, "高标液5启用"=0, "低斜率"=0.0, "低截距"=0.0, "低二次多项式系数"=0.0, "低线性相关系数"=0.0, "高斜率"=0.0, "高截距"=0.0, "高二次多项式系数"=0.0, "高线性相关系数"=0.0}, "校准信息改变"=FALSE, "固件版本号"=""}  # 与CODCr交互全局
      n42 = Obtain Queue(name (unnamed)="CODCr interface Read" ("写入方名称"), element data type=w68) -> (queue out=w69:refnum<queue>)  [unwired: 3 in, 2 out]
    }
  }
  n43 = case shown="True" w1 {
    tunnel: [_ w72] -> w35
    tunnel: [_ w71] -> w34
    frame False {
    }
    frame True {
      w71 = T10 {"状态告警区"={"系统时间"=timestamp(0 s since 1904-01-01), "工作状态"=0, "测量模式"=enum."待机", "告警代码"=0, "故障代码"=0, "日志代码"=0, "软件版本"=0, "F0"=0.0, "F1"=0.0, "F2"=0.0, "F3"=0.0, "T"=0.0, "H"=0.0, "id"=0, "flowid"=0, "量程"=0, "总磷控温温度1"=0.0, "营养盐控温温度2"=0.0, "ADC"=0.0}, "平台试剂余量百分比"=0.0, "关键参数"={"测量量程"=0.0, "测量精度"=0.0, "测量间隔"=0.0, "消解温度"=0.0, "消解时长"=0.0, "空白校准时间"=timestamp(0 s since 1904-01-01), "曲线截距"=0.0, "曲线斜率"=0.0, "测量检出限"=0.0, "测量信号值"=0.0, "线性相关系数"=0.0, "二次多项式系数"=0.0, "标样校准时间"=timestamp(0 s since 1904-01-01), "稀释倍数"=0.0, "三项式系数"=0.0, "空白标定系数"=0.0, "量程系数"=0.0, "F0/ORPA"=0.0, "F1/ORPB"=0.0, "F2/ORPK"=0.0, "F3"=0.0, "F4"=0.0, "F5"=0.0, "F6"=0.0, "F7"=0.0, "X0/滴定数"=0.0, "量程"=0.0}, "关键参数改变"=FALSE, "校准信息"={"低标液1浓度"=0.0, "低标液1信号值"=0.0, "低标液1启用"=0, "低标液2浓度"=0.0, "低标液2信号值"=0.0, "低标液2启用"=0, "低标液3浓度"=0.0, "低标液3信号值"=0.0, "低标液3启用"=0, "低标液4浓度"=0.0, "低标液4信号值"=0.0, "低标液4启用"=0, "低标液5浓度"=0.0, "低标液5信号值"=0.0, "低标液5启用"=0, "高标液1浓度"=0.0, "高标液1信号值"=0.0, "高标液1启用"=0, "高标液2浓度"=0.0, "高标液2信号值"=0.0, "高标液2启用"=0, "高标液3浓度"=0.0, "高标液3信号值"=0.0, "高标液3启用"=0, "高标液4浓度"=0.0, "高标液4信号值"=0.0, "高标液4启用"=0, "高标液5浓度"=0.0, "高标液5信号值"=0.0, "高标液5启用"=0, "低斜率"=0.0, "低截距"=0.0, "低二次多项式系数"=0.0, "低线性相关系数"=0.0, "高斜率"=0.0, "高截距"=0.0, "高二次多项式系数"=0.0, "高线性相关系数"=0.0}, "校准信息改变"=FALSE, "固件版本号"=""}  # 与CODMn交互全局
      n44 = Obtain Queue(name (unnamed)="CODMn interface Read" ("写入方名称"), element data type=w71) -> (queue out=w72:refnum<queue>)  [unwired: 3 in, 2 out]
    }
  }
  n45 = case shown="True" w5 {
    tunnel: [_ w75] -> w27
    tunnel: [_ w74] -> w26
    frame False {
    }
    frame True {
      w74 = T11 {"状态告警区"={"系统时间"=timestamp(0 s since 1904-01-01), "工作状态"=0, "测量模式"=enum."待机", "告警代码"=0, "故障代码"=0, "日志代码"=0, "软件版本"=0, "F0"=0.0, "F1"=0.0, "F2"=0.0, "F3"=0.0, "T"=0.0, "H"=0.0, "id"=0, "flowid"=0, "量程"=0, "总磷控温温度1"=0.0, "营养盐控温温度2"=0.0, "ADC"=0.0}, "平台试剂余量百分比"=0.0, "关键参数"={"测量量程"=0.0, "测量精度"=0.0, "测量间隔"=0.0, "消解温度"=0.0, "消解时长"=0.0, "空白校准时间"=timestamp(0 s since 1904-01-01), "曲线截距"=0.0, "曲线斜率"=0.0, "测量检出限"=0.0, "测量信号值"=0.0, "线性相关系数"=0.0, "二次多项式系数"=0.0, "标样校准时间"=timestamp(0 s since 1904-01-01), "稀释倍数"=0.0, "三项式系数"=0.0, "空白标定系数"=0.0, "量程系数"=0.0, "F0/ORPA"=0.0, "F1/ORPB"=0.0, "F2/ORPK"=0.0, "F3"=0.0, "F4"=0.0, "F5"=0.0, "F6"=0.0, "F7"=0.0, "X0/滴定数"=0.0, "量程"=0.0}, "关键参数改变"=FALSE, "校准信息"={"低标液1浓度"=0.0, "低标液1信号值"=0.0, "低标液1启用"=0, "低标液2浓度"=0.0, "低标液2信号值"=0.0, "低标液2启用"=0, "低标液3浓度"=0.0, "低标液3信号值"=0.0, "低标液3启用"=0, "低标液4浓度"=0.0, "低标液4信号值"=0.0, "低标液4启用"=0, "低标液5浓度"=0.0, "低标液5信号值"=0.0, "低标液5启用"=0, "高标液1浓度"=0.0, "高标液1信号值"=0.0, "高标液1启用"=0, "高标液2浓度"=0.0, "高标液2信号值"=0.0, "高标液2启用"=0, "高标液3浓度"=0.0, "高标液3信号值"=0.0, "高标液3启用"=0, "高标液4浓度"=0.0, "高标液4信号值"=0.0, "高标液4启用"=0, "高标液5浓度"=0.0, "高标液5信号值"=0.0, "高标液5启用"=0, "低斜率"=0.0, "低截距"=0.0, "低二次多项式系数"=0.0, "低线性相关系数"=0.0, "高斜率"=0.0, "高截距"=0.0, "高二次多项式系数"=0.0, "高线性相关系数"=0.0}, "校准信息改变"=FALSE, "固件版本号"=""}  # 与氨氮交互全局
      n46 = Obtain Queue(name (unnamed)="氨氮 interface Read" ("写入方名称"), element data type=w74) -> (queue out=w75:refnum<queue>)  [unwired: 3 in, 2 out]
    }
  }
  n47 = case shown="True" w4 {
    tunnel: [_ w78] -> w29
    tunnel: [_ w77] -> w28
    frame False {
    }
    frame True {
      w77 = T12 {"状态告警区"={"系统时间"=timestamp(0 s since 1904-01-01), "工作状态"=0, "测量模式"=enum."待机", "告警代码"=0, "故障代码"=0, "日志代码"=0, "软件版本"=0, "F0"=0.0, "F1"=0.0, "F2"=0.0, "F3"=0.0, "T"=0.0, "H"=0.0, "id"=0, "flowid"=0, "量程"=0, "总磷控温温度1"=0.0, "营养盐控温温度2"=0.0, "ADC"=0.0}, "平台试剂余量百分比"=0.0, "关键参数"={"测量量程"=0.0, "测量精度"=0.0, "测量间隔"=0.0, "消解温度"=0.0, "消解时长"=0.0, "空白校准时间"=timestamp(0 s since 1904-01-01), "曲线截距"=0.0, "曲线斜率"=0.0, "测量检出限"=0.0, "测量信号值"=0.0, "线性相关系数"=0.0, "二次多项式系数"=0.0, "标样校准时间"=timestamp(0 s since 1904-01-01), "稀释倍数"=0.0, "三项式系数"=0.0, "空白标定系数"=0.0, "量程系数"=0.0, "F0/ORPA"=0.0, "F1/ORPB"=0.0, "F2/ORPK"=0.0, "F3"=0.0, "F4"=0.0, "F5"=0.0, "F6"=0.0, "F7"=0.0, "X0/滴定数"=0.0, "量程"=0.0}, "关键参数改变"=FALSE, "校准信息"={"低标液1浓度"=0.0, "低标液1信号值"=0.0, "低标液1启用"=0, "低标液2浓度"=0.0, "低标液2信号值"=0.0, "低标液2启用"=0, "低标液3浓度"=0.0, "低标液3信号值"=0.0, "低标液3启用"=0, "低标液4浓度"=0.0, "低标液4信号值"=0.0, "低标液4启用"=0, "低标液5浓度"=0.0, "低标液5信号值"=0.0, "低标液5启用"=0, "高标液1浓度"=0.0, "高标液1信号值"=0.0, "高标液1启用"=0, "高标液2浓度"=0.0, "高标液2信号值"=0.0, "高标液2启用"=0, "高标液3浓度"=0.0, "高标液3信号值"=0.0, "高标液3启用"=0, "高标液4浓度"=0.0, "高标液4信号值"=0.0, "高标液4启用"=0, "高标液5浓度"=0.0, "高标液5信号值"=0.0, "高标液5启用"=0, "低斜率"=0.0, "低截距"=0.0, "低二次多项式系数"=0.0, "低线性相关系数"=0.0, "高斜率"=0.0, "高截距"=0.0, "高二次多项式系数"=0.0, "高线性相关系数"=0.0}, "校准信息改变"=FALSE, "固件版本号"=""}  # 与总氮交互全局
      n48 = Obtain Queue(name (unnamed)="总氮 interface Read" ("写入方名称"), element data type=w77) -> (queue out=w78:refnum<queue>)  [unwired: 3 in, 2 out]
    }
  }
  n49 = case shown="True" w3 {
    tunnel: [_ w81] -> w31
    tunnel: [_ w80] -> w30
    frame False {
    }
    frame True {
      w80 = T13 {"状态告警区"={"系统时间"=timestamp(0 s since 1904-01-01), "工作状态"=0, "测量模式"=enum."待机", "告警代码"=0, "故障代码"=0, "日志代码"=0, "软件版本"=0, "F0"=0.0, "F1"=0.0, "F2"=0.0, "F3"=0.0, "T"=0.0, "H"=0.0, "id"=0, "flowid"=0, "量程"=0, "总磷控温温度1"=0.0, "营养盐控温温度2"=0.0, "ADC"=0.0}, "平台试剂余量百分比"=0.0, "关键参数"={"测量量程"=0.0, "测量精度"=0.0, "测量间隔"=0.0, "消解温度"=0.0, "消解时长"=0.0, "空白校准时间"=timestamp(0 s since 1904-01-01), "曲线截距"=0.0, "曲线斜率"=0.0, "测量检出限"=0.0, "测量信号值"=0.0, "线性相关系数"=0.0, "二次多项式系数"=0.0, "标样校准时间"=timestamp(0 s since 1904-01-01), "稀释倍数"=0.0, "三项式系数"=0.0, "空白标定系数"=0.0, "量程系数"=0.0, "F0/ORPA"=0.0, "F1/ORPB"=0.0, "F2/ORPK"=0.0, "F3"=0.0, "F4"=0.0, "F5"=0.0, "F6"=0.0, "F7"=0.0, "X0/滴定数"=0.0, "量程"=0.0}, "关键参数改变"=FALSE, "校准信息"={"低标液1浓度"=0.0, "低标液1信号值"=0.0, "低标液1启用"=0, "低标液2浓度"=0.0, "低标液2信号值"=0.0, "低标液2启用"=0, "低标液3浓度"=0.0, "低标液3信号值"=0.0, "低标液3启用"=0, "低标液4浓度"=0.0, "低标液4信号值"=0.0, "低标液4启用"=0, "低标液5浓度"=0.0, "低标液5信号值"=0.0, "低标液5启用"=0, "高标液1浓度"=0.0, "高标液1信号值"=0.0, "高标液1启用"=0, "高标液2浓度"=0.0, "高标液2信号值"=0.0, "高标液2启用"=0, "高标液3浓度"=0.0, "高标液3信号值"=0.0, "高标液3启用"=0, "高标液4浓度"=0.0, "高标液4信号值"=0.0, "高标液4启用"=0, "高标液5浓度"=0.0, "高标液5信号值"=0.0, "高标液5启用"=0, "低斜率"=0.0, "低截距"=0.0, "低二次多项式系数"=0.0, "低线性相关系数"=0.0, "高斜率"=0.0, "高截距"=0.0, "高二次多项式系数"=0.0, "高线性相关系数"=0.0}, "校准信息改变"=FALSE, "固件版本号"=""}  # 与总磷交互全局
      n50 = Obtain Queue(name (unnamed)="总磷 interface Read" ("写入方名称"), element data type=w80) -> (queue out=w81:refnum<queue>)  [unwired: 3 in, 2 out]
    }
  }
  n51 = Obtain Queue(name (unnamed)=w36, element data type=w41) -> (queue out=w37:refnum<queue>, error out=w40:errorcluster)  [unwired: 3 in, 1 out]
  n52 = while {
    tunnel: w7 -> [w87]
    tunnel: w6 -> [w86]
    tunnel: [w85] -> _
    tunnel: [w84] -> _
    stop <- FALSE stop-if-true
    n53 = for {
      tunnel: w87 -> [w94] mode=indexing
      tunnel: w86 -> [w93] mode=indexing
      tunnel: [w92] -> w85
      tunnel: [w91] -> w84
      n54 = Dequeue Element(queue=w94, timeout in ms (-1)=1000 ("超时毫秒(-1)"), error in (no error)=w93) -> (queue out=w92:refnum<queue>, element=w90:cluster{"selected path":path}, timed out?=w88:bool, error out=w91:errorcluster)
      n55 = case shown="False" w88 {
        tunnel: w90 -> [w103 _]
        frame False {
          n56 = Unbundle By Name(w103) -> ("selected path"=w102:path)
          n57 = call "固件升级（包含参数恢复）.vi"("路径对话框"=FALSE, "selected path"=w102) -> ("结果字符串"=w96:string)  [unwired: 9 in]
          n58 = global read "VAR总磷总氮全局变量.vi" "模块名称"() -> (w98:string)
          n59 = Concatenate Strings("平台反控固件升级" ("日志信息"), w96) -> (w95:string)
          n60 = Get Date/Time In Seconds() -> (seconds since 1Jan1904=w99:timestamp)
          n61 = Bundle By Name(cluster=T14 {"时间"=timestamp(0 s since 1904-01-01), "参数"="", "日志信息"="", "流程参数"=""} ("data in"), "时间"=w99, "参数"=w98, "日志信息"=w95) -> (w100:T14)
          n62 = call "总磷总氮操作日志.vi"("data in"=w100) -> ()  [unwired: 10 in, 1 out]
        }
        frame True {
        }
      }
    }
  }
  n63 = Generate Occurrence() -> (w38:refnum<k4>)
  n64 = while {
    tunnel: w37 -> [w107]
    tunnel: w38 -> [w105]
    stop <- w106 stop-if-true
    n65 = event shown="[3] \"启动\": Value Change" {
      selector: _ -> [_ _ _ _ _ _ _ _]
      dyn-events: _ -> [_ _ _ _ _ _ _ _]
      timeout: _ -> [_ _ _ _ _ _ _ _]
      tunnel: w107 -> [_ _ _ w139 w149 w155 w160 w165]
      tunnel: [_ _ _ _ "停止" _ _ _] -> w106
      tunnel: w105 -> [_ _ _ _ w146 _ _ _]
      event Timeout {
        n66 = event-data() -> ()  [unwired: 1 in, 3 out]
      }
      event "启用模块": Value Change {
        n67 = event-data() -> ("NewVal"=w108:bool)  [unwired: 1 in, 5 out]
        n68 = call <vilib>:"Application Directory.vi"() -> ("Application Directory"=w110:path)
        n69 = Build Path(base path=w110, name or relative path="data\\set.ini" ("名称或相对路径")) -> (appended path=w111:path)
        n70 = call <vilib>:"Open Config Data.vi"("configuration file path"=w111) -> ("error out"=w117:errorcluster, "refnum"=w116:T15)  [unwired: 8 in, 1 out]
        n71 = call-poly <vilib>:"Write Key.vi"("section"="总磷总氮", "error in (no error)"=w117, "value"=w108, "key"="模块启用", "refnum"=w116) -> ("error out"=w113:errorcluster, "refnum out"=w109:T15)  [unwired: 4 in, 1 out]
        n72 = call <vilib>:"Close Config Data.vi"("error in (no error)"=w113, "refnum"=w109) -> ()  [unwired: 8 in, 2 out]
      }
      event "VISA Resource": Value Change {
        n73 = event-data() -> ()  [unwired: 1 in, 6 out]
        n74 = call <vilib>:"Application Directory.vi"() -> ("Application Directory"=w120:path)
        n75 = Build Path(base path=w120, name or relative path="data\\set.ini" ("名称或相对路径")) -> (appended path=w121:path)
        n76 = call <vilib>:"Open Config Data.vi"("configuration file path"=w121) -> ("error out"=w127:errorcluster, "refnum"=w126:T15)  [unwired: 8 in, 1 out]
        n77 = call-poly <vilib>:"Write Key.vi"("section"="总磷总氮", "error in (no error)"=w127, "value"="VISA Resource", "key"="串口", "refnum"=w126) -> ("error out"=w123:errorcluster, "refnum out"=w119:T15)  [unwired: 4 in, 1 out]
        n78 = call <vilib>:"Close Config Data.vi"("error in (no error)"=w123, "refnum"=w119) -> ()  [unwired: 8 in, 2 out]
      }
      event "启动": Value Change {
        n79 = event-data() -> ()  [unwired: 1 in, 6 out]
        n80 = global read "总磷总氮断电保存全局变量.vi" "协议"() -> (w130:u16)
        n81 = case shown="0, Default" w130 {
          tunnel: "控制命令" -> [w140 w142]
          tunnel: [w140 w141] -> w128
          frame 0, Default {
          }
          frame 1 {
            n82 = Swap Bytes(anything=w142) -> (byte swapped=w141:u16)
          }
        }
        n83 = case shown="Default" "控制命令" {
          tunnel: "控制命令参数" -> [w144 w145]
          tunnel: [w143 w145] -> w131
          frame Default {
            n84 = call "HexToWord.vi"("数组"=w144) -> ("WORD"=w143:u16[])  [unwired: 10 in]
          }
          frame 13 {
          }
        }
        n85 = call "控制命令区.vi"("控制命令参数"=w131, "控制命令"=w128) -> ("控制命令"=w135:u16[])  [unwired: 9 in]
        n86 = local read "站号"() -> (w134:u16)
        n87 = Bundle("站号"=w134, "控制命令"=w135) -> (w133:cluster{"站号":u16, "控制命令":u16[]})  [unwired: 1 in]
        n88 = Bundle By Name(cluster=cluster{"命令":string, "data":variant} {"命令"="", "data"=variant} ("元素"), "命令"="启动", "data"=w133) -> (w137:cluster{"命令":string, "data":variant})
        n89 = Enqueue Element(queue=w139, element=w137) -> ()  [unwired: 2 in, 3 out]
      }
      event "停止": Value Change {
        n90 = event-data() -> ()  [unwired: 1 in, 6 out]
        n91 = Set Occurrence(w146) -> ()
        n92 = Flush Queue(queue=w149) -> (queue out=w148:refnum<queue>)  [unwired: 1 in, 2 out]
        n93 = Enqueue Element(queue=w148, element=cluster{"命令":string, "data":variant} {"命令"="shutdown", "data"=variant} ("元素")) -> ()  [unwired: 2 in, 3 out]
      }
      event "读测量数据区": Value Change {
        n94 = event-data() -> ()  [unwired: 1 in, 6 out]
        n95 = Bundle By Name(cluster=cluster{"命令":string, "data":variant} {"命令"="", "data"=variant} ("元素"), "命令"="读测量数据区", "data"="站号") -> (w153:cluster{"命令":string, "data":variant})
        n96 = Enqueue Element(queue=w155, element=w153) -> ()  [unwired: 2 in, 3 out]
      }
      event "读状态告警区": Value Change {
        n97 = event-data() -> ()  [unwired: 1 in, 6 out]
        n98 = local read "站号"() -> (w156:u16)
        n99 = Bundle By Name(cluster=cluster{"命令":string, "data":variant} {"命令"="", "data"=variant} ("元素"), "命令"="读状态告警区", "data"=w156) -> (w158:cluster{"命令":string, "data":variant})
        n100 = Enqueue Element(queue=w160, element=w158) -> ()  [unwired: 2 in, 3 out]
      }
      event "读关键参数区": Value Change {
        n101 = event-data() -> ()  [unwired: 1 in, 6 out]
        n102 = local read "站号"() -> (w161:u16)
        n103 = Bundle By Name(cluster=cluster{"命令":string, "data":variant} {"命令"="", "data"=variant} ("元素"), "命令"="读关键参数区", "data"=w161) -> (w163:cluster{"命令":string, "data":variant})
        n104 = Enqueue Element(queue=w165, element=w163) -> ()  [unwired: 2 in, 3 out]
      }
    }
  }
  n105 = while {
    tunnel: w38 -> [w176]
    tunnel: w37 -> [w172]
    stop <- w173 stop-if-true
    n106 = global read "总磷总氮断电保存全局变量.vi" "MB通信方式选择"() -> (w171:enum16{"串口", "TCP"})
    n107 = Wait on Occurrence(2:w176, 3:10000 ("毫秒超时(-1)")) -> (0:w174:bool)  [unwired: 1 in]
    n108 = Not(x=w174) -> (.not. x?=w173:bool)
    n109 = case shown="\"TCP\"" w171 {
      tunnel: [_ w177] -> w168
      frame "串口", Default {
      }
      frame "TCP" {
        n110 = global read "VAR总磷总氮全局变量.vi" "MB session in"() -> (w179:refnum<class "MB_Master.lvclass">)
        n111 = property class="MB_Master"(reference=w179) -> ("Properties:Session Valid"=w178:bool)  [unwired: 1 in, 2 out]
        n112 = Not(x=w178) -> (.not. x?=w177:bool)
      }
    }
    n113 = First Call?() -> (First Call?: T/F=w170:bool)
    n114 = Or(x=w168, y=w170) -> (x .or. y?=w169:bool)
    n115 = local read "启用"() -> (w166:bool)
    n116 = And(x=w166, y=w169) -> (x .and. y?=w167:bool)
    n117 = case shown="True" w167 {
      tunnel: w172 -> [_ w182]
      frame False {
      }
      frame True {
        n118 = Flush Queue(queue=w182) -> (queue out=w180:refnum<queue>)  [unwired: 1 in, 2 out]
        n119 = Enqueue Element(queue=w180, element=cluster{"命令":string, "data":variant} {"命令"="启用模块", "data"=variant} ("元素")) -> ()  [unwired: 2 in, 3 out]
        n120 = property on="VISA Resource" class="VISAName"("DisabledEnum"=T16."Disabled and Grayed Out" ("禁用")) -> ()  [unwired: 2 in, 2 out]
      }
    }
  }
  n121 = while {
    tunnel: w37 -> [w200]
    tunnel: w40 -> [w199]
    shift-right: [w187] -> _
    shift-left: _ -> [w197]
    tunnel: errorcluster {"status"=FALSE, "code"=0, "source"=""} ("error out") -> [w196]
    tunnel: [w184] -> _
    stop <- w198 stop-if-true
    n122 = Dequeue Element(queue=w200, error in (no error)=w199) -> (queue out=w193:refnum<queue>, element=w194:cluster{"命令":string, "data":variant})  [unwired: 1 in, 2 out]
    n123 = Unbundle By Name(w194) -> ("命令"=w195:string, "data"=w191:variant)
    n124 = case shown="\"读测量数据区\"" w195 {
      tunnel: w191 -> [_ _ _ w238 w252 w269 w277 w402 w462 _]
      tunnel: w193 -> [_ _ _ _ _ _ w278 _ _ w475]
      tunnel: [_ _ _ _ _ _ _ _ _ TRUE] -> w198
      tunnel: [w203 w206 w224 w241 w255 w271 w299 w410 w469 w471] -> w187
      tunnel: [w204 w205 w225 w240 w254 w270 w300 w401 w470 w472] -> w184
      tunnel: w197 -> [w203 _ w224 w237 w251 w268 w295 w405 w465 w471]
      tunnel: w196 -> [w204 _ w226 w234 w248 w265 w293 w406 w466 w473]
      tunnel: [_ _ _ w229 w245 w259 w273 w383 w456 _] -> w185
      frame Default {
      }
      frame "启用模块" {
        n125 = global read "总磷总氮断电保存全局变量.vi" "MB通信方式选择"() -> (w207:enum16{"串口", "TCP"})
        n126 = case shown="\"串口\", Default" w207 {
          tunnel: [w215 w220] -> w205
          tunnel: [w212 w219] -> w206
          frame "串口", Default {
            n127 = global read "总磷总氮断电保存全局变量.vi" "波特率"() -> (w210:u32)
            n128 = Bundle By Name(cluster=T17 {"baud rate (bps)"=115200, "stop bits"=10, "parity"=0, "flow control"=0, "timeout"=1000, "retries"=1} ("Serial Config"), "baud rate (bps)"=w210) -> (w209:T17)
            n129 = global read "总磷总氮断电保存全局变量.vi" "VISA Resource"() -> (w213:refnum<visa-resource-name>)
            n130 = call <vilib>:"Open Serial Session.vi"("Mode (RTU)"=enum16{"RTU", "ASCII"}."RTU", "Slave ID"=u8 1, "Serial Config"=w209, "VISA Resource"=w213) -> ("Error out"=w215:errorcluster, "MB_Serial session"=w212:refnum<class "MB_Master_Serial.lvclass">)  [unwired: 6 in]
          }
          frame "TCP" {
            n131 = global read "总磷总氮断电保存全局变量.vi" "PORT"() -> (w218:string)
            n132 = Decimal String To Number(string=w218) -> (number=w221:i32)  [unwired: 2 in, 1 out]
            n133 = global read "总磷总氮断电保存全局变量.vi" "IP"() -> (w217:string)
            n134 = call <vilib>:"Open TCP Session.vi"("Port (502)"=w221, "IP Address"=w217) -> ("error out"=w220:errorcluster, "MB_TCP session"=w219:refnum<class "MB_Master_TCP.lvclass">)  [unwired: 8 in]
          }
        }
        "启用" <- TRUE
      }
      frame "停用模块" {
        n135 = call-dynamic "Close Session.vi"("error in (no error)"=w226, "MB session in"=w224) -> ("error out"=w222:errorcluster)  [unwired: 9 in]
        n136 = local write "启用"(FALSE ("启用")) -> ()
        n137 = call <vilib>:"Clear Errors.vi"("error in (no error)"=w222) -> ("error out"=w225:errorcluster)  [unwired: 5 in, 1 out]
      }
      frame "启动" {
        n138 = Variant To Data(type=cluster{"站号":u16, "控制命令":u16[]} {"站号"=0, "控制命令"=[]} ("输出簇"), Variant=w238) -> (data=w232:cluster{"站号":u16, "控制命令":u16[]})  [unwired: 1 in, 1 out]
        n139 = Unbundle By Name(w232) -> ("站号"=w229:u16, "控制命令"=w230:u16[])
        n140 = property class="MB_Master"(reference=w237, error in=w234, "Properties:Slave ID"=w229) -> (reference out=w236:refnum<class "MB_Master.lvclass">, error out=w235:errorcluster)
        n141 = Index Array(array=w230) -> (element=w231:u16)  [unwired: 1 in]
        n142 = global read "总磷总氮断电保存全局变量.vi" "波特率"() -> (w227:u32)
        n143 = case shown="9600" w227 {
          tunnel: w231 -> [w242 w244]
          tunnel: [w242 w243] -> w228
          frame 9600 {
          }
          frame 115200, Default {
            n144 = Swap Bytes(anything=w244) -> (byte swapped=w243:u16)
          }
        }
        n145 = call <vilib>:"Write Multiple Registers.vi"("error in (no error)"=w235, "values"=w230, "starting address"=u16 4608, "MB session in"=w236) -> ("error out"=w240:errorcluster, "MB session out"=w241:refnum<class "MB_Master.lvclass">)  [unwired: 6 in]
        n146 = global write "VAR总磷总氮全局变量.vi" "控制命令"(w228) -> ()
      }
      frame "盲样测试" {
        n147 = Variant To Data(type=u8 0, Variant=w252) -> (data=w245:u8)  [unwired: 1 in, 1 out]
        n148 = property class="MB_Master"(reference=w251, error in=w248, "Properties:Slave ID"=w245) -> (reference out=w250:refnum<class "MB_Master.lvclass">, error out=w249:errorcluster)
        n149 = case shown="Default" w245 {
          tunnel: [u16[] [] ("values") u16[] [33539, 0] ("values") u16[] [23555, 0] ("values")] -> w247
          frame Default {
          }
          frame 1 {
            # "总磷盲样测试命令"
          }
          frame 3 {
            # "氨氮盲样测试"
          }
        }
        n150 = call <vilib>:"Write Multiple Registers.vi"("error in (no error)"=w249, "values"=w247, "starting address"=u16 24592, "MB session in"=w250) -> ("error out"=w254:errorcluster, "MB session out"=w255:refnum<class "MB_Master.lvclass">)  [unwired: 6 in]
      }
      frame "debug" {
        n151 = Variant To Data(type=cluster{"站号":u16, "控制命令":u16[]} {"站号"=0, "控制命令"=[]} ("输出簇"), Variant=w269) -> (data=w263:cluster{"站号":u16, "控制命令":u16[]})  [unwired: 1 in, 1 out]
        n152 = Unbundle By Name(w263) -> ("站号"=w259:u16, "控制命令"=w261:u16[])
        n153 = property class="MB_Master"(reference=w268, error in=w265, "Properties:Slave ID"=w259) -> (reference out=w267:refnum<class "MB_Master.lvclass">, error out=w266:errorcluster)
        n154 = Index Array(array=w261) -> (element=w262:u16)  [unwired: 1 in]
        n155 = global write "VAR总磷总氮全局变量.vi" "控制命令"(w262) -> ()
        n156 = call <vilib>:"Write Multiple Registers.vi"("error in (no error)"=w266, "values"=w261, "starting address"=u16 24594, "MB session in"=w267) -> ("error out"=w270:errorcluster, "MB session out"=w271:refnum<class "MB_Master.lvclass">)  [unwired: 6 in]
      }
      frame "读测量数据区" {
        n157 = global read "model config var.vi" "启动队列名称"() -> (w275:cluster{"String":string, "Value":u16}[])
        n158 = Bundle("命令"="读关键参数区", "data"=w277) -> (w279:cluster{"命令":string, "data":variant})  [unwired: 1 in]
        n159 = Variant To Data(type=u8 1 ("Slave ID"), Variant=w277) -> (data=w273:u8)  [unwired: 1 in, 1 out]
        n160 = property class="MB_Master"(reference=w295, error in=w293, "Properties:Slave ID"=w273) -> (reference out=w294:refnum<class "MB_Master.lvclass">, error out=w292:errorcluster)
        n161 = Enqueue Element(queue=w278, element=w279) -> ()  [unwired: 2 in, 3 out]
        n162 = Index Array(array=w275) -> (element=w276:cluster{"String":string, "Value":u16})  [unwired: 1 in]
        n163 = Unbundle By Name(w276) -> ("Value"=w274:u16)
        n164 = global read "VAR总磷总氮全局变量.vi" "测量数据区数组"() -> (w289:T8)
        n165 = Not Equal?(x=w274, y=w273) -> (x != y?=w272:bool)
        n166 = call "id参数转换.vi"("id"=w274) -> ("数组资源索引"=w284:i32)  [unwired: 9 in, 1 out]
        n167 = call <vilib>:"Read Holding Registers.vi"("error in (no error)"=w292, "quantity"=u16 107, "starting address"=u16 4096, "MB session in"=w294) -> ("error out"=w300:errorcluster, "Registers"=w291:u16[], "MB session out"=w299:refnum<class "MB_Master.lvclass">)  [unwired: 5 in]
        n168 = call "id参数转换.vi"("id"=w273) -> ("数组资源索引"=w285:i32)  [unwired: 9 in, 1 out]
        n169 = Index Array(array=w289, index #1=w285, index #2=w284) -> (element #1=w290:T5, element #2=w286:T5)
        n170 = call "测量数据区_选择.vi"("data"=w291) -> ("测量数据区"=w281:T5)  [unwired: 10 in]
        "测量数据区" <- w281
        n171 = global write "VAR总磷总氮全局变量.vi" "测量数据区"(w281) -> ()
        n172 = global read "工况数据接口全局.vi" "data"() -> (w283:T18)
        n173 = case shown="22" w273 {
          selector: w273 -> [w306 _ _ _ _]
          tunnel: w281 -> [w303 w348 w357 w370 w377]
          tunnel: w291 -> [_ w351 w369 w376 w382]
          tunnel: w290 -> [w305 w341 _ _ _]
          tunnel: [w301 w350 w357 w370 w377] -> w288
          tunnel: w286 -> [w304 w340 _ _ _]
          tunnel: w283 -> [w307 w349 w368 w375 w381]
          tunnel: [w307 w342 w358 w371 w380] -> w282
          tunnel: w272 -> [w302 w339 _ _ _]
          frame 0, Default {
            n174 = case shown="0, Default" w306 {
              tunnel: w305 -> [_ w313 w323 w333]
              tunnel: w304 -> [_ w312 w322 w332]
              tunnel: w303 -> [w308 w311 w321 w331]
              tunnel: w302 -> [_ w310 w320 w330]
              tunnel: [w308 w309 w319 w329] -> w301
              frame 0, Default {
              }
              frame 4 {
                n175 = case shown="True" w310 {
                  tunnel: w313 -> [w314 w318]
                  tunnel: w312 -> [_ w317]
                  tunnel: w311 -> [_ w316]
                  tunnel: [w314 w315] -> w309
                  frame False {
                  }
                  frame True {
                    # "非首参自动对齐"
                    n176 = call "数据时间对齐.vi"("待对齐时间"=w316, "对齐参考时间"=w317, "已对齐时间输入"=w318) -> ("已对齐时间输出"=w315:T5)  [unwired: 8 in]
                  }
                }
              }
              frame 5 {
                n177 = case shown="True" w320 {
                  tunnel: w323 -> [w324 w328]
                  tunnel: w322 -> [_ w327]
                  tunnel: w321 -> [_ w326]
                  tunnel: [w324 w325] -> w319
                  frame False {
                  }
                  frame True {
                    # "非首参自动对齐"
                    n178 = call "数据时间对齐.vi"("待对齐时间"=w326, "对齐参考时间"=w327, "已对齐时间输入"=w328) -> ("已对齐时间输出"=w325:T5)  [unwired: 8 in]
                  }
                }
              }
              frame 6 {
                n179 = case shown="True" w330 {
                  tunnel: w333 -> [w334 w338]
                  tunnel: w332 -> [_ w337]
                  tunnel: w331 -> [_ w336]
                  tunnel: [w334 w335] -> w329
                  frame False {
                  }
                  frame True {
                    # "非首参自动对齐"
                    n180 = call "数据时间对齐.vi"("待对齐时间"=w336, "对齐参考时间"=w337, "已对齐时间输入"=w338) -> ("已对齐时间输出"=w335:T5)  [unwired: 8 in]
                  }
                }
              }
            }
          }
          frame 1 {
            n181 = Unbundle By Name(w348) -> ("F0"=w347:sgl, "F1"=w346:sgl, "F2"=w345:sgl, "F3"=w344:sgl, "X值"=w343:sgl)
            n182 = case shown="True" w339 {
              tunnel: [w352 w356] -> w350
              tunnel: w341 -> [_ w355]
              tunnel: w340 -> [_ w354]
              tunnel: w348 -> [w352 w353]
              frame False {
              }
              frame True {
                # "启动总磷总氮时间自动对齐"
                n183 = call "数据时间对齐.vi"("待对齐时间"=w353, "对齐参考时间"=w354, "已对齐时间输入"=w355) -> ("已对齐时间输出"=w356:T5)  [unwired: 8 in]
              }
            }
            n184 = Bundle By Name(cluster=w349, "data.TP.TP.F0"=w347, "data.TP.TP.F1"=w346, "data.TP.TP.F2"=w345, "data.TP.TP.F3"=w344, "data.TP.TP.X0"=w343) -> (w342:T18)
            "总磷测量数据区" <- w351
          }
          frame 2 {
            n185 = Unbundle By Name(w357) -> ("F0"=w367:sgl, "F1"=w366:sgl, "F2"=w365:sgl, "F3"=w364:sgl, "F4"=w363:sgl, "F5"=w362:sgl, "F6"=w361:sgl, "F7"=w360:sgl, "X值"=w359:sgl)
            n186 = Bundle By Name(cluster=w368, "data.TN.TN.F0"=w367, "data.TN.TN.F1"=w366, "data.TN.TN.F2"=w365, "data.TN.TN.F3"=w364, "data.TN.TN.F4"=w363, "data.TN.TN.F5"=w362, "data.TN.TN.F6"=w361, "data.TN.TN.F7"=w360, "data.TN.TN.X0"=w359) -> (w358:T18)
            "总氮测量数据区" <- w369
          }
          frame 3 {
            n187 = Unbundle By Name(w370) -> ("F0"=w374:sgl, "F1"=w373:sgl, "X值"=w372:sgl)
            n188 = Bundle By Name(cluster=w375, "data.NH3.NH3.F0"=w374, "data.NH3.NH3.F1"=w373, "data.NH3.NH3.X0"=w372) -> (w371:T18)
            "氨氮测量数据区" <- w376
          }
          frame 22 {
            n189 = Unbundle By Name(w377) -> ("F0"=w379:sgl, "F1"=w378:sgl)
            n190 = Bundle By Name(cluster=w381, "data.CODCr.CODCr.F0"=w379, "data.CODCr.CODCr.F1"=w378) -> (w380:T18)
            "COD测量数据区" <- w382
          }
        }
        n191 = global write "工况数据接口全局.vi" "data"(w282) -> ()
        n192 = Replace Array Subset(array=w289, new element=w288, index=w285) -> (w287:T8)
        n193 = global write "VAR总磷总氮全局变量.vi" "测量数据区数组"(w287) -> ()
      }
      frame "读状态告警区" {
        n194 = Variant To Data(type=u8 1 ("Slave ID"), Variant=w402) -> (data=w383:u8)  [unwired: 1 in, 1 out]
        n195 = property class="MB_Master"(reference=w405, error in=w406, "Properties:Slave ID"=w383) -> (reference out=w404:refnum<class "MB_Master.lvclass">, error out=w403:errorcluster)
        n196 = call "id参数转换.vi"("id"=w383) -> ("数组资源索引"=w396:i32)  [unwired: 9 in, 1 out]
        n197 = call <vilib>:"Read Holding Registers.vi"("error in (no error)"=w403, "quantity"=u16 44, "starting address"=u16 4224, "MB session in"=w404) -> ("error out"=w401:errorcluster, "Registers"=w399:u16[], "MB session out"=w410:refnum<class "MB_Master.lvclass">)  [unwired: 5 in]
        n198 = global read "VAR总磷总氮全局变量.vi" "状态告警区数组"() -> (w398:T7)
        n199 = call "状态告警区_选择.vi"("Slave ID"=w383, "data"=w399) -> ("状态告警区 2"=w384:T19, "状态告警区"=w385:T4)  [unwired: 8 in]
        "状态告警区" <- w384
        n200 = Unbundle By Name(w385) -> ("日志代码"=w386:u16, "告警代码"=w392:u16, "故障代码"=w390:u16)
        n201 = global write "VAR总磷总氮全局变量.vi" "状态告警区"(w384) -> ()
        n202 = Unbundle By Name(w385) -> ("id"=w400:u16)
        n203 = Replace Array Subset(array=w398, new element=w385, index=w396) -> (w397:T7)
        n204 = global write "VAR总磷总氮全局变量.vi" "状态告警区数组"(w397) -> ()
        n205 = feedback-in #1(w392) -> ()
        n206 = feedback #1() -> (w393:u16)  [unwired: 1 in]
        n207 = feedback #2() -> (w391:u16)  [unwired: 1 in]
        n208 = feedback-in #2(w390) -> ()
        n209 = Not Equal?(x=w393, y=w392) -> (x != y?=w389:bool)
        n210 = Not Equal?(x=w391, y=w390) -> (x != y?=w388:bool)
        n211 = Or(x=w389, y=w388) -> (x .or. y?=w387:bool)
        n212 = global read "工况数据接口全局.vi" "data"() -> (w395:T18)
        n213 = case shown="1, 131" w400 {
          tunnel: w385 -> [_ w423 w436 w446 w452]
          tunnel: w399 -> [_ w424 w437 w447 w454]
          tunnel: w395 -> [w411 w414 w429 w442 w453]
          tunnel: [w411 w421 w431 w445 w450] -> w394
          tunnel: w387 -> [_ w416 w427 w441 _]
          tunnel: w386 -> [_ w415 w426 w440 _]
          frame 0, Default {
          }
          frame 1, 131 {
            n214 = Unbundle By Name(w414) -> ("data.TP.TP.alarm_step"=w413:dbl)
            n215 = Unbundle By Name(w423) -> ("总磷控温温度1"=w422:sgl, "营养盐控温温度2"=w418:sgl)
            n216 = Select(t=w415, s=w416, f=w413) -> (s? t:f=w412:dbl)
            n217 = global read "VAR总磷总氮全局变量.vi" "总磷关键参数"() -> (w420:T20)
            n218 = Unbundle By Name(w420) -> ("消解温度"=w419:sgl)
            n219 = Bundle By Name(cluster=w414, "data.TP.TP.alarm_step"=w412, "data.TP.TP.digestion_temperature"=w422, "data.TP.TP.constant_temperature"=w419, "data.TP.TP.syringe_temperature"=w418, "data.TP.启用"=TRUE) -> (w421:T18)
            "总磷状态告警区" <- w424
          }
          frame 2, 76 {
            n220 = Unbundle By Name(w429) -> ("data.TN.TN.alarm_step"=w428:dbl)
            n221 = Unbundle By Name(w436) -> ("总磷控温温度1"=w432:sgl, "营养盐控温温度2"=w434:sgl)
            n222 = Select(t=w426, s=w427, f=w428) -> (s? t:f=w425:dbl)
            n223 = global read "VAR总磷总氮全局变量.vi" "总氮关键参数"() -> (w435:T20)
            n224 = Unbundle By Name(w435) -> ("消解温度"=w433:sgl)
            n225 = Bundle By Name(cluster=w429, "data.TN.TN.alarm_step"=w425, "data.TN.TN.digestion_temperature"=w432, "data.TN.TN.constant_temperature"=w433, "data.TN.TN.syringe_temperature"=w434, "data.TN.启用"=TRUE) -> (w431:T18)
            "总氮状态告警区" <- w437
          }
          frame 3 {
            n226 = Unbundle By Name(w442) -> ("data.NH3.NH3.alarm_step"=w439:dbl)
            n227 = Unbundle By Name(w446) -> ("营养盐控温温度2"=w444:sgl)
            n228 = Select(t=w440, s=w441, f=w439) -> (s? t:f=w438:dbl)
            n229 = Bundle By Name(cluster=w442, "data.NH3.NH3.alarm_step"=w438, "data.NH3.NH3.syringe_temperature"=w444, "data.NH3.启用"=TRUE) -> (w445:T18)
            "氨氮状态告警区" <- w447
          }
          frame 22 {
            n230 = Unbundle By Name(w452) -> ("营养盐控温温度2"=w451:sgl)
            n231 = global read "VAR总磷总氮全局变量.vi" "波形图-消解温度"() -> (w448:sgl[])
            n232 = Bundle By Name(cluster=w453, "data.CODCr.CODCr.temperature_curve"=w448, "data.CODCr.CODCr.reagent_sensor"=w451, "data.CODCr.启用"=TRUE) -> (w450:T18)
            "COD状态告警区" <- w454
          }
        }
        n233 = global write "工况数据接口全局.vi" "data"(w394) -> ()
      }
      frame "读关键参数区" {
        n234 = Variant To Data(type=u8 1 ("Slave ID"), Variant=w462) -> (data=w456:u8)  [unwired: 1 in, 1 out]
        n235 = property class="MB_Master"(reference=w465, error in=w466, "Properties:Slave ID"=w456) -> (reference out=w464:refnum<class "MB_Master.lvclass">, error out=w463:errorcluster)
        n236 = call "id参数转换.vi"("id"=w456) -> ("数组资源索引"=w455:i32)  [unwired: 9 in, 1 out]
        n237 = call <vilib>:"Read Holding Registers.vi"("error in (no error)"=w463, "quantity"=u16 56, "starting address"=u16 4256, "MB session in"=w464) -> ("error out"=w470:errorcluster, "Registers"=w460:u16[], "MB session out"=w469:refnum<class "MB_Master.lvclass">)  [unwired: 5 in]
        n238 = global read "VAR总磷总氮全局变量.vi" "关键参数区数组"() -> (w459:T6)
        n239 = call "关键参数区.vi"("数组"=w460) -> ("关键参数区"=w458:T3)  [unwired: 10 in]
        "关键参数区" <- w458
        n240 = global write "VAR总磷总氮全局变量.vi" "关键参数区"(w458) -> ()
        n241 = Replace Array Subset(array=w459, new element=w458, index=w455) -> (w457:T6)
        n242 = global write "VAR总磷总氮全局变量.vi" "关键参数区数组"(w457) -> ()
      }
      frame "shutdown" {
        n243 = call-dynamic "Close Session.vi"("error in (no error)"=w473, "MB session in"=w471) -> ("error out"=w472:errorcluster)  [unwired: 9 in]
        n244 = Flush Queue(queue=w475) -> (queue out=w474:refnum<queue>)  [unwired: 1 in, 2 out]
        n245 = Release Queue(queue=w474) -> ()  [unwired: 2 in, 3 out]
      }
    }
    n246 = global write "VAR总磷总氮全局变量.vi" "MB session in"(w187) -> ()
    n247 = Unbundle By Name(w184) -> ("status"=w190:bool)
    n248 = Not(x=w190) -> (.not. x?=w192:bool)
    "status" <- w192
    n249 = call <vilib>:"Boolean Crossing PtByPt.vi"("direction"=enum16{"either", "false-true", "true-false"}."false-true", "input"=w190) -> ("crossing"=w189:bool)  [unwired: 1 in]
    n250 = case shown="False" w189 {
      tunnel: [u16 0 ("告警代码") u16 999 ("告警代码")] -> w186
      frame False {
      }
      frame True {
      }
    }
    n251 = global write "VAR总磷总氮全局变量.vi" "通讯状态"(w192) -> ()
    n252 = call "告警码字段定义.vi"("id"=w185, "告警代码"=w186) -> ()  [unwired: 9 in, 1 out]
  }
  n253 = while {
    tunnel: w35 -> [w487]
    tunnel: w34 -> [w486]
    tunnel: w33 -> [w485]
    tunnel: w32 -> [w484]
    tunnel: w31 -> [w483]
    tunnel: w30 -> [w482]
    tunnel: w29 -> [w481]
    tunnel: w28 -> [w480]
    tunnel: w27 -> [w479]
    tunnel: w26 -> [w478]
    stop <- FALSE stop-if-true
    n254 = global read "model config var.vi" "启动队列名称"() -> (w490:cluster{"String":string, "Value":u16}[])
    n255 = Wait (ms)(milliseconds to wait=u32 1000 ("等待时间（毫秒）")) -> ()  [unwired: 1 out]
    n256 = global read "VAR总磷总氮全局变量.vi" "固件版本号"() -> (w477:string)
    n257 = for {
      tunnel: w490 -> [w503] mode=indexing
      tunnel: w487 -> [w501]
      tunnel: w486 -> [w500]
      tunnel: w485 -> [w499]
      tunnel: w484 -> [w498]
      tunnel: w483 -> [w497]
      tunnel: w482 -> [w496]
      tunnel: w481 -> [w495]
      tunnel: w480 -> [w494]
      tunnel: w479 -> [w493]
      tunnel: w478 -> [w492]
      tunnel: w477 -> [w491]
      n258 = Unbundle By Name(w503) -> ("Value"=w502:u16)
      n259 = case shown="21" w502 {
        tunnel: w501 -> [_ _ _ _ w590 _]
        tunnel: w500 -> [_ _ _ _ w589 _]
        tunnel: w499 -> [_ _ _ w569 _ _]
        tunnel: w498 -> [_ _ _ w568 _ _]
        tunnel: w497 -> [w506 _ _ _ _ _]
        tunnel: w496 -> [w505 _ _ _ _ _]
        tunnel: w495 -> [_ w527 _ _ _ _]
        tunnel: w494 -> [_ w526 _ _ _ _]
        tunnel: w493 -> [_ _ w548 _ _ _]
        tunnel: w492 -> [_ _ w547 _ _ _]
        tunnel: w491 -> [w504 w525 w546 w567 w588 _]
        frame 1 {
          n260 = Get Queue Status(queue=w506) -> (queue out=w509:refnum<queue>, # elements in queue=w508:i32)  [unwired: 2 in, 6 out]
          n261 = Equal To 0?(x=w508) -> (x = 0?=w507:bool)
          n262 = case shown="True" w507 {
            tunnel: w505 -> [_ w521]
            tunnel: w509 -> [_ w522]
            tunnel: w504 -> [_ w510]
            frame False {
            }
            frame True {
              w512 = u16 1 items=["总磷"=1, "总氮"=2, "氨氮"=3, "磷酸盐"=4, "硝氮"=5, "亚硝氮"=6, "硅酸盐"=7, "硫化物"=8, "CODCr"=22]
              n263 = Unbundle By Name(w521) -> ("关键参数"=w519:T21)
              n264 = global read "VAR总磷总氮全局变量.vi" "总磷关键参数"() -> (w520:T20)
              n265 = global read "VAR总磷总氮全局变量.vi" "状态告警区数组"() -> (w514:T7)
              n266 = global read "VAR总磷总氮全局变量.vi" "平台试剂余量百分比"() -> (w524:sgl)
              n267 = call "id参数转换.vi"("id"=w512) -> ("数组资源索引"=w513:i32)  [unwired: 9 in, 1 out]
              n268 = call "转换关键参数(子VI).vi"("参数"=w512, "总磷关键参数"=w520, "关键参数输入"=w519) -> ("关键参数输出"=w518:T21)  [unwired: 8 in]
              n269 = global read "VAR总磷总氮全局变量.vi" "总磷关键参数改变"() -> (w517:bool)
              n270 = global read "VAR总磷总氮全局变量.vi" "总磷校准信息改变"() -> (w515:bool)
              n271 = global read "VAR总磷总氮全局变量.vi" "总磷校准信息"() -> (w516:T22)
              n272 = Index Array(array=w514, index=w513) -> (element=w511:T4)
              n273 = Bundle By Name(cluster=w521, "状态告警区"=w511, "平台试剂余量百分比"=w524, "关键参数"=w518, "关键参数改变"=w517, "校准信息"=w516, "校准信息改变"=w515, "固件版本号"=w510) -> (w523:T13)
              n274 = Enqueue Element(queue=w522, element=w523) -> ()  [unwired: 2 in, 3 out]
            }
          }
        }
        frame 2 {
          n275 = Get Queue Status(queue=w527) -> (queue out=w530:refnum<queue>, # elements in queue=w529:i32)  [unwired: 2 in, 6 out]
          n276 = Equal To 0?(x=w529) -> (x = 0?=w528:bool)
          n277 = case shown="True" w528 {
            tunnel: w530 -> [_ w543]
            tunnel: w526 -> [_ w541]
            tunnel: w525 -> [_ w531]
            frame False {
            }
            frame True {
              w533 = u16 2 items=["总磷"=1, "总氮"=2, "氨氮"=3, "磷酸盐"=4, "硝氮"=5, "亚硝氮"=6, "硅酸盐"=7, "硫化物"=8, "CODCr"=22]
              n278 = Unbundle By Name(w541) -> ("关键参数"=w540:T21)
              n279 = global read "VAR总磷总氮全局变量.vi" "总氮关键参数"() -> (w542:T20)
              n280 = global read "VAR总磷总氮全局变量.vi" "状态告警区数组"() -> (w534:T7)
              n281 = global read "VAR总磷总氮全局变量.vi" "平台试剂余量百分比"() -> (w545:sgl)
              n282 = call "id参数转换.vi"("id"=w533) -> ("数组资源索引"=w535:i32)  [unwired: 9 in, 1 out]
              n283 = call "转换关键参数(子VI).vi"("参数"=w533, "总磷关键参数"=w542, "关键参数输入"=w540) -> ("关键参数输出"=w539:T21)  [unwired: 8 in]
              n284 = global read "VAR总磷总氮全局变量.vi" "总氮关键参数改变"() -> (w538:bool)
              n285 = global read "VAR总磷总氮全局变量.vi" "总氮校准信息改变"() -> (w536:bool)
              n286 = global read "VAR总磷总氮全局变量.vi" "总氮校准信息"() -> (w537:T22)
              n287 = Index Array(array=w534, index=w535) -> (element=w532:T4)
              n288 = Bundle By Name(cluster=w541, "状态告警区"=w532, "平台试剂余量百分比"=w545, "关键参数"=w539, "关键参数改变"=w538, "校准信息"=w537, "校准信息改变"=w536, "固件版本号"=w531) -> (w544:T12)
              n289 = Enqueue Element(queue=w543, element=w544) -> ()  [unwired: 2 in, 3 out]
            }
          }
        }
        frame 3 {
          (unwired) FALSE
          n290 = Get Queue Status(queue=w548) -> (queue out=w550:refnum<queue>, # elements in queue=w551:i32)  [unwired: 2 in, 6 out]
          n291 = Equal To 0?(x=w551) -> (x = 0?=w549:bool)
          n292 = case shown="True" w549 {
            tunnel: w550 -> [_ w564]
            tunnel: w547 -> [_ w563]
            tunnel: w546 -> [_ w552]
            frame False {
            }
            frame True {
              w554 = u16 3 items=["总磷"=1, "总氮"=2, "氨氮"=3, "磷酸盐"=4, "硝氮"=5, "亚硝氮"=6, "硅酸盐"=7, "硫化物"=8, "CODCr"=22]
              n293 = Unbundle By Name(w563) -> ("关键参数"=w562:T21)
              n294 = global read "VAR总磷总氮全局变量.vi" "氨氮关键参数"() -> (w560:T20)
              n295 = global read "VAR总磷总氮全局变量.vi" "状态告警区数组"() -> (w555:T7)
              n296 = global read "VAR总磷总氮全局变量.vi" "平台试剂余量百分比"() -> (w566:sgl)
              n297 = call "id参数转换.vi"("id"=w554) -> ("数组资源索引"=w556:i32)  [unwired: 9 in, 1 out]
              n298 = call "转换关键参数(子VI).vi"("参数"=w554, "总磷关键参数"=w560, "关键参数输入"=w562) -> ("关键参数输出"=w561:T21)  [unwired: 8 in]
              n299 = global read "VAR总磷总氮全局变量.vi" "氨氮关键参数改变"() -> (w559:bool)
              n300 = global read "VAR总磷总氮全局变量.vi" "氨氮校准信息改变"() -> (w557:bool)
              n301 = global read "VAR总磷总氮全局变量.vi" "氨氮校准信息"() -> (w558:T22)
              n302 = Index Array(array=w555, index=w556) -> (element=w553:T4)
              n303 = Bundle By Name(cluster=w563, "状态告警区"=w553, "平台试剂余量百分比"=w566, "关键参数"=w561, "关键参数改变"=w559, "校准信息"=w558, "校准信息改变"=w557, "固件版本号"=w552) -> (w565:T11)
              n304 = Enqueue Element(queue=w564, element=w565) -> ()  [unwired: 2 in, 3 out]
            }
          }
        }
        frame 22 {
          n305 = Get Queue Status(queue=w569) -> (queue out=w571:refnum<queue>, # elements in queue=w572:i32)  [unwired: 2 in, 6 out]
          n306 = Equal To 0?(x=w572) -> (x = 0?=w570:bool)
          n307 = case shown="True" w570 {
            tunnel: w571 -> [_ w585]
            tunnel: w568 -> [_ w584]
            tunnel: w567 -> [_ w573]
            frame False {
            }
            frame True {
              w575 = u16 22 items=["总磷"=1, "总氮"=2, "氨氮"=3, "磷酸盐"=4, "硝氮"=5, "亚硝氮"=6, "硅酸盐"=7, "硫化物"=8, "CODCr"=22]
              n308 = Unbundle By Name(w584) -> ("关键参数"=w583:T21)
              n309 = global read "VAR总磷总氮全局变量.vi" "CODcr关键参数"() -> (w582:T20)
              n310 = global read "VAR总磷总氮全局变量.vi" "状态告警区数组"() -> (w576:T7)
              n311 = global read "VAR总磷总氮全局变量.vi" "CODCr关键参数改变"() -> (w580:bool)
              n312 = global read "VAR总磷总氮全局变量.vi" "CODCr校准信息改变"() -> (w578:bool)
              n313 = global read "VAR总磷总氮全局变量.vi" "平台试剂余量百分比"() -> (w587:sgl)
              n314 = call "id参数转换.vi"("id"=w575) -> ("数组资源索引"=w577:i32)  [unwired: 9 in, 1 out]
              n315 = call "转换关键参数(子VI).vi"("参数"=w575, "总磷关键参数"=w582, "关键参数输入"=w583) -> ("关键参数输出"=w581:T21)  [unwired: 8 in]
              n316 = global read "VAR总磷总氮全局变量.vi" "CODCr校准信息"() -> (w579:T22)
              n317 = Index Array(array=w576, index=w577) -> (element=w574:T4)
              n318 = Bundle By Name(cluster=w584, "状态告警区"=w574, "平台试剂余量百分比"=w587, "关键参数"=w581, "关键参数改变"=w580, "校准信息"=w579, "校准信息改变"=w578, "固件版本号"=w573) -> (w586:T10)
              n319 = Enqueue Element(queue=w585, element=w586) -> ()  [unwired: 2 in, 3 out]
            }
          }
        }
        frame 21 {
          (unwired) FALSE
          n320 = Get Queue Status(queue=w590) -> (queue out=w592:refnum<queue>, # elements in queue=w593:i32)  [unwired: 2 in, 6 out]
          n321 = Equal To 0?(x=w593) -> (x = 0?=w591:bool)
          n322 = case shown="True" w591 {
            tunnel: w592 -> [_ w606]
            tunnel: w589 -> [_ w605]
            tunnel: w588 -> [_ w594]
            frame False {
            }
            frame True {
              w596 = u16 21 items=["总磷"=1, "总氮"=2, "氨氮"=3, "磷酸盐"=4, "硝氮"=5, "亚硝氮"=6, "硅酸盐"=7, "硫化物"=8, "CODMn"=21, "CODCr"=22, "氟化物"=50]
              n323 = Unbundle By Name(w605) -> ("关键参数"=w604:T21)
              n324 = global read "VAR总磷总氮全局变量.vi" "CODMn关键参数"() -> (w603:T20)
              n325 = global read "VAR总磷总氮全局变量.vi" "状态告警区数组"() -> (w597:T7)
              n326 = global read "VAR总磷总氮全局变量.vi" "CODmn关键参数改变"() -> (w601:bool)
              n327 = global read "VAR总磷总氮全局变量.vi" "CODMn校准信息改变"() -> (w599:bool)
              n328 = global read "VAR总磷总氮全局变量.vi" "平台试剂余量百分比"() -> (w608:sgl)
              n329 = call "id参数转换.vi"("id"=w596) -> ("数组资源索引"=w598:i32)  [unwired: 9 in, 1 out]
              n330 = call "转换关键参数(子VI).vi"("参数"=w596, "总磷关键参数"=w603, "关键参数输入"=w604) -> ("关键参数输出"=w602:T21)  [unwired: 8 in]
              n331 = global read "VAR总磷总氮全局变量.vi" "CODMn校准信息"() -> (w600:T22)
              n332 = Index Array(array=w597, index=w598) -> (element=w595:T4)
              n333 = Bundle By Name(cluster=w605, "状态告警区"=w595, "平台试剂余量百分比"=w608, "关键参数"=w602, "关键参数改变"=w601, "校准信息"=w600, "校准信息改变"=w599, "固件版本号"=w594) -> (w607:T10)
              n334 = Enqueue Element(queue=w606, element=w607) -> ()  [unwired: 2 in, 3 out]
            }
          }
        }
        frame Default {
        }
      }
    }
  }
